vi "Station Detail Main.vi"(8 "error in (no error)":errorcluster, 11 "NG Pick in":refnum<class "NG Pick.lvclass">) -> (0 "error out":errorcluster, 2 "Station Out":T1=enum."ImformOut", 3 "NG Pick out":refnum<class "NG Pick.lvclass">)   [LabVIEW 2019, in "NG Pick.lvclass"]
uses:
  NG Pick.lvclass
  Ctrl/Station Action.ctl
  Ctrl/ProjectStepSelect.ctl
  Ctrl/StationCmdSelect.ctl
  Ctrl/Auto Inspection Station Name2.ctl
  Ctrl/Auto Inspection Data Name.ctl
  Ctrl/MeasureDisplayTab.ctl
  Ctrl/Table Save.ctl
  Ctrl/S2 Station IO.ctl
  Ctrl/ModbusCmd.ctl
  Ctrl/S2 Station Input.ctl
  Global/Process Global.vi
  LLB/Commonly VI/Main Glb.vi
  Ctrl/ProjectCmdStep.ctl
  LineScan/LineScan.lvclass
  LLB/Commonly VI.lvlib
  Ctrl/PD Table Save Low Index.ctl
  Ctrl/PD Table Save Col Index.ctl
panel:
  out "Array":string[](array[string])
  out "Blue Scan receive":string
  out "S1 ChkSum":string
  out "S1 ToolStringOut":string
  out "ToolStringOut_P1_2":string
  out "P1 Receive":string[](array[string])
  out "ToolStringOut_P1":string
  out "ToolStringOut_Init":string
  out "Initial_ChkSum":string
  out "Initial receive 2":string
  in  "Table Control":string[][](table)=[["PCBA BARCODE", ""], ["硬體(Tool初始化)", ""], ["company(Tool初始化)", ""], ["耗電流 uA(電流表)", "T"], ["電池負載電壓", "T"], ["晶片ID(Tool FORMAT)", "F"], ["雷雕ID(TOOl scan、藍芽接收器)", "S"], ["Format(Tool FORMAT)", "F"], ["Programe(Tool Programe)", "P"]]
  out "Numeric":dbl
  out "subarray":string[](array[string])
  out "T2 buffer":string
  out "T1 buffer":string
  out "S2 receive":string
  out "Blue Scan2 receive":string
  out "Program receive":string
  out "format receive":string
  out "Initial receive":string
  out "present":i32
  out "Retry":i32
  out "Act Step":i32
  out "retry次數":string[](array[string])
  out "CurrentCmd":string
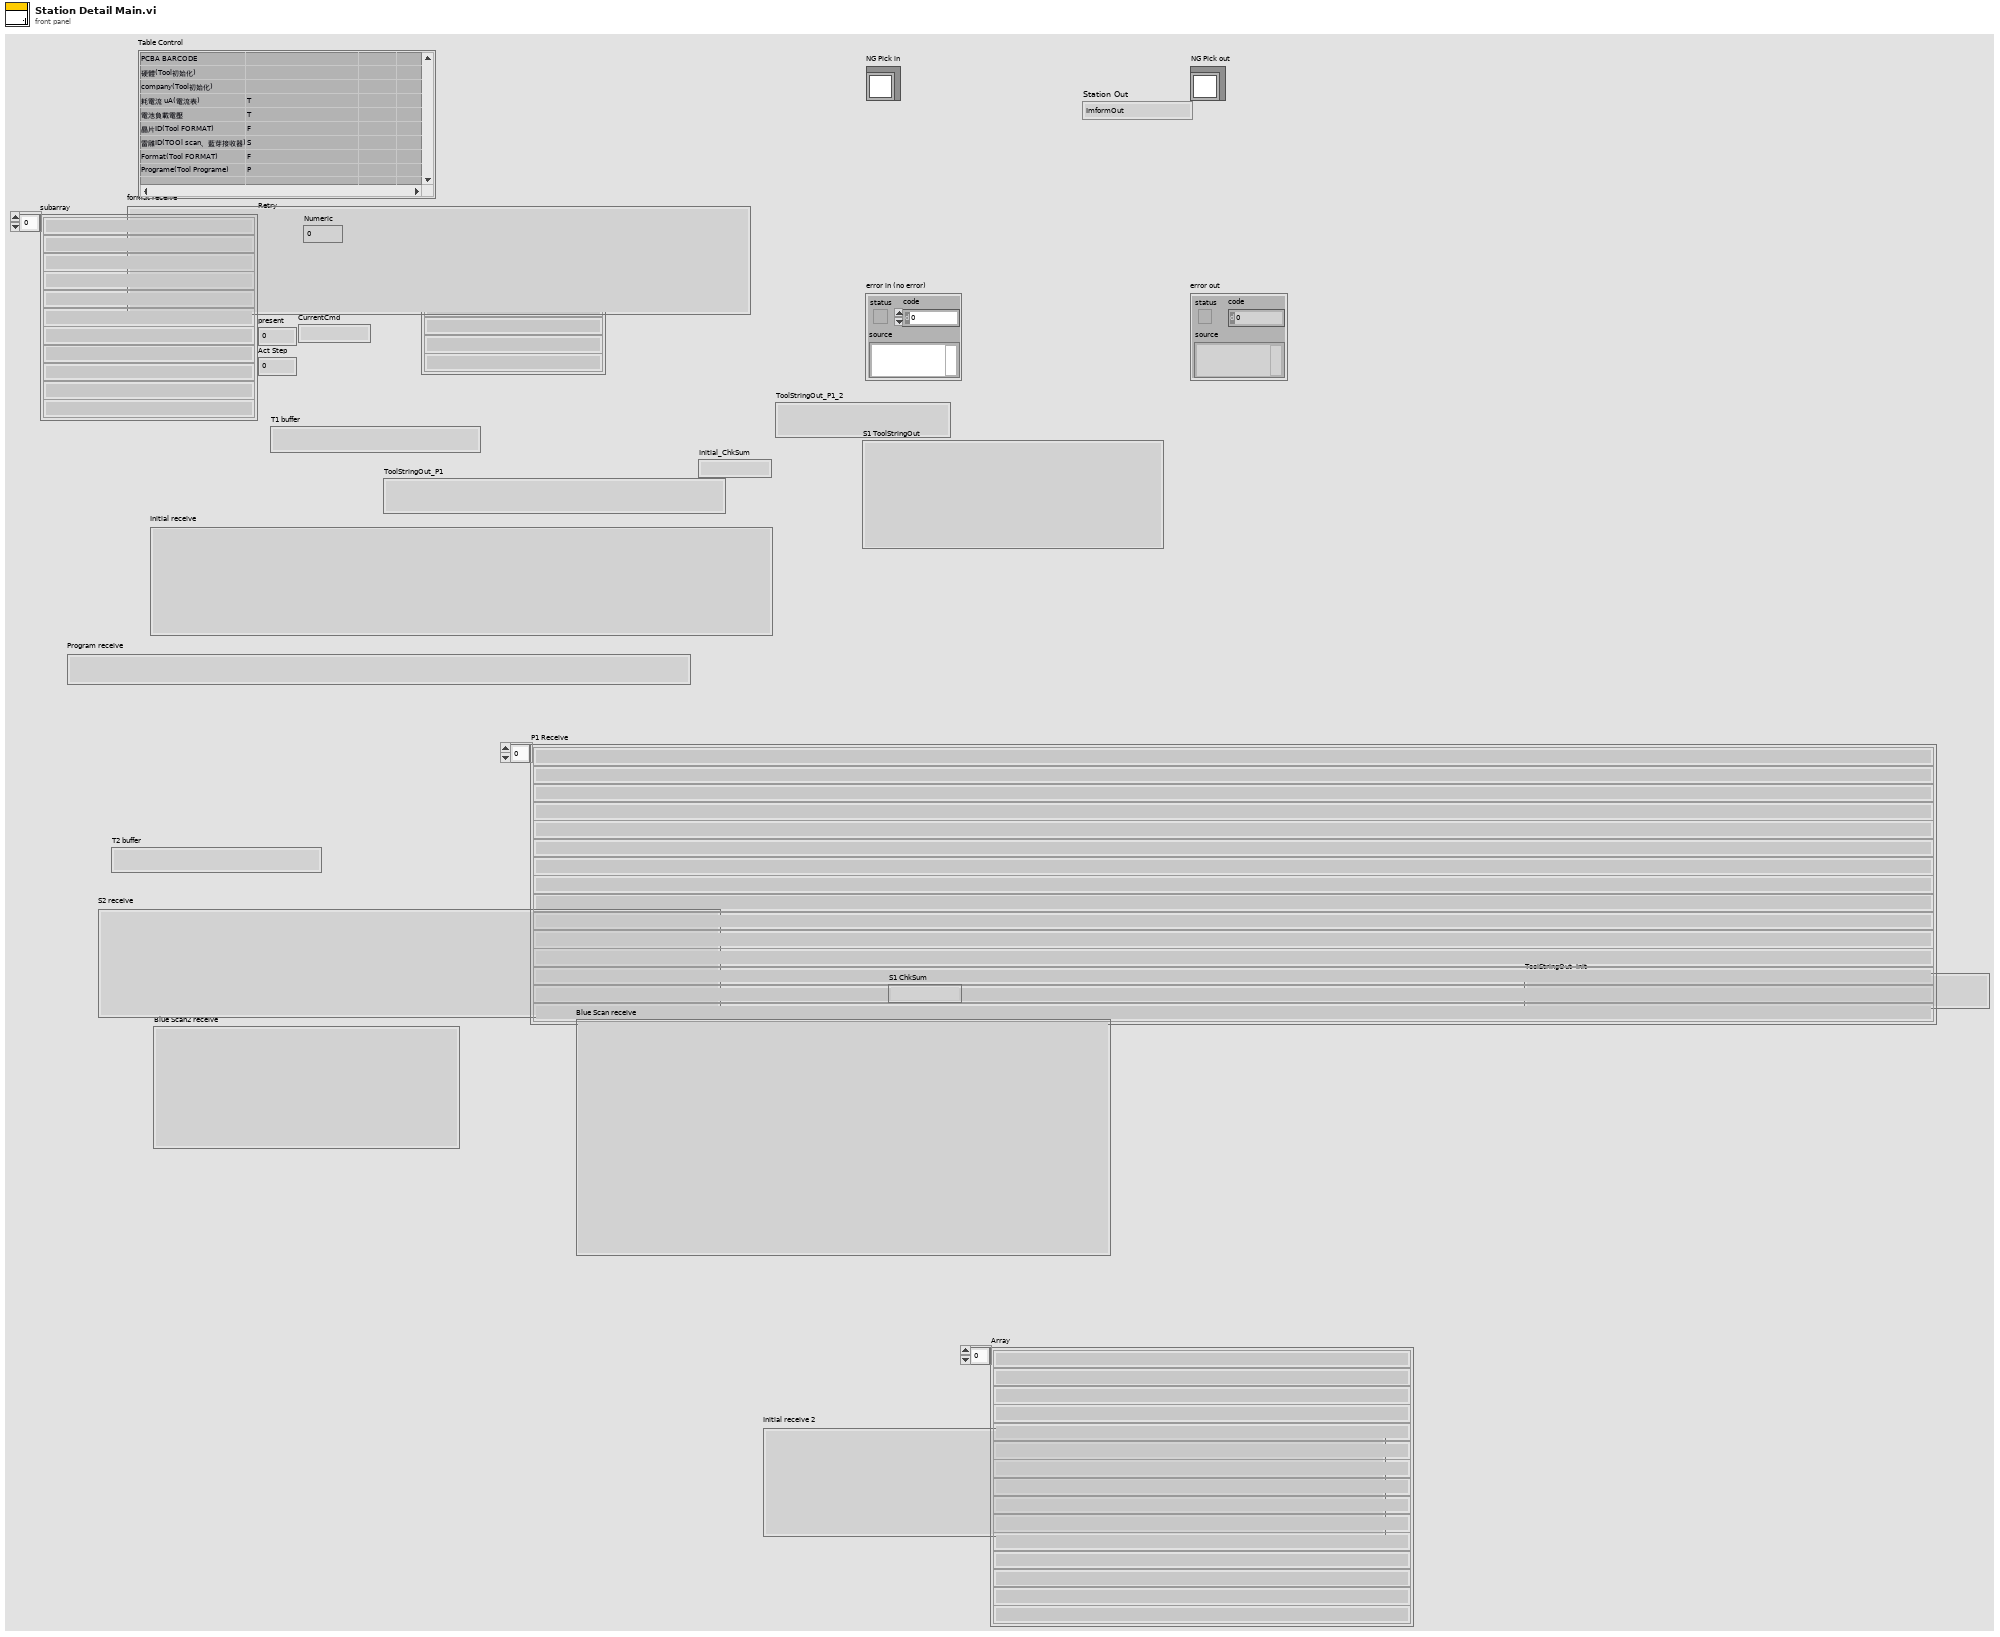
[diagram p1: front panel]
types:
  T1 = typedef "Station Action.ctl" = enum16{"Wait Item In", "Dectect Action", "ImformOut"}
  T2 = typedef "StationCmdSelect.ctl" = enum16{"Action", "Command", "Return", "DTime", "Retry"}
  T3 = typedef "Auto Inspection Data Name.ctl" = enum16{"LocalRun", "ItemSN(TimeCode)", "CurrentAction", "Error", "Data", "OKNG", "電壓值", "電壓值判斷", "電流值", "電流值判斷", "Laser1 Data", "Laser2 Data", "Laser OKNG", "StationNO"}
  T4 = typedef "Auto Inspection Station Name2.ctl" = enum16{"S1Barcode", "S2Measure", "S3Measure", "S4Measure", "S5Measure", "S11_LaserCheck", "S8_Vision AI"}
  T5 = typedef "Table Save.ctl" = enum16{"initial", "Add", "Write", "Replace", "Delete", "REad", "RedTable", "Load"}
  T6 = typedef "MeasureDisplayTab.ctl" = enum16{"Tray Barcode", "PCBA BARCODE", "硬體(Tool初始化)", "company(Tool初始化)", "耗電流 uA(電流表)", "電池負載電壓", "晶片ID(Tool FORMAT)", "雷雕ID(TOOl scan、藍芽接收器)", "Format(Tool FORMAT)", "Programe(Tool Programe)", "MAC(藍芽接收器)", "ID(藍芽接收器)", "KPA(藍芽接收器)", "溫度(藍芽接收器)", "SENSOR電池電壓(藍芽接收器)", "RSSI(藍芽接收器)", "SensorType_315(FSK scan)", "FSKsnVol_315(FSK scan)", "FSKscanl_315(FSK scan)", "P_315(FSK scan)", "T_315(FSK scan)", "SensorType_433(ASK scan)", "ASKsnVol_433(ASK scan)", "ASKscan_433(ASK scan)", "P_433(ASK scan)", "T_433(ASK scan)", "測高Data"}
  T7 = typedef "PD Table Save Col Index.ctl" = enum16{"Col A", "Col B", "PCBA SN_C", "scan 半成品 ID_1_D", "半成品 Waste_Time_E", "半成品 Result_F", "半成品 DateTime_G", "433半成品 版本_H", "433半成品 company_I", "433半成品 FF_J", "433半成品 SensorType_K", "433半成品 BattVol_L", "433半成品 ASKsnVOL_M", "433半成品 ID_2_N", "433半成品 Format_O", "433半成品 Programe_P", "433半成品 ASKscan_Q", "433半成品 FSKscan_R", "433半成品 Batt_S", "433半成品 SN_T", "433半成品 Ptest_U", "433半成品 Ttest_V", "433半成品 P_W", "433半成品 T_X", "433半成品 結果_Y", "433半成品 箱號_Z", "不良代碼_AA", "電流_AB", "電池電壓_AC", "315半成品 版本_AD", "315半成品 company_AE", "315半成品 FF_AF", "315半成品 SensorType_AG", "315半成品 BattVol_AH", "315半成品 ASKsnVOL_AI", "315半成品 ID_2_AJ", "315半成品 Format_AK", "315半成品 Programe_AL", "315半成品 ASKscan_AM", "315半成品 FSKscan_AN", "315半成品 Batt_AO", "315半成品 SN_AP", "315半成品 Ptest_AQ", "315半成品 Ttest_AR", "315半成品 P_AS", "315半成品 T_AT"}
  T8 = typedef "PD Table Save Low Index.ctl" = enum16{"low 1", "low 2", "low 3", "low 4", "一般模式F", "一般模式P", "一般模式S", "low 8", "藍芽模式F", "藍芽模式P", "藍芽模式S"}
  T9 = cluster{"starting address":u16, "number of inputs":u16, "Sat Coils":bool[], "Holding Registers":u16[]}
  T10 = typedef "ModbusCmd.ctl" = enum16{"Connect", "Disconnect", "Init", "Fetch Basic Objects", "Fetch Input Refisters", "Fetch Discrete Inputs", "Set Coils", "Set Holding Registers", "Write Single Holding", "Exit"}
  T11 = typedef "S2 Station Input.ctl" = enum16{"00PLC Alive clock", "01PLC狀態(手動)", "02PLC狀態(自動)", "03PLC Alarm", "04備用", "05備用", "06備用", "07備用", "08備用", "09備用", "10載盤有料for條碼", "11_備用", "12_備用", "13_備用", "14_備用", "15_備用", "16_備用", "17_備用", "18_備用", "19_備用", "20_載盤有料訊號ForS2站", "21_PLC下達可測電流訊號", "22_PLC下達可測電壓訊號"}
  T12 = typedef "ProjectStepSelect.ctl" = enum16{"ProjectName", "Name", "Initial", "Reset", "Format", "Program1", "Program2", "Scan", "Finish", "MToolWork", "DataCheck", "DataSave", "OutputPLC", "WaitInputS1", "WaitInputOff"}
  T13 = typedef "S2 Station IO.ctl" = enum16{"S2站PC動作中_20", "電流量測完成產品OK_21", "電流量測完成產品NG_22", "S2站Format 執行_23", "S2 Format OK_24", "S2 Format NG_25", "S2站燒入執行_26", "S2站燒入OK_27", "S2站燒入NG_28", "S2站動作完成_29", "S3 PC動作中_30", "S3 Format 此站執行_31", "S3 Format OK_32", "S3 Format NG_33", "S3 燒入程式 此站執行_34", "S3 燒入程式 OK_35", "S3 燒入程式 NG_36", "S3 備用_37", "S3 備用_38", "S3 動作完成_39", "S4 PC動作中_40", "S4 量測完成 產品正常_41", "S4 量測完成 產品NG_42", "S4 Format 此站執行_43", "S4 Format OK_44", "S4 Format NG_45", "S4 燒入 此站不執行_46", "S4 燒入程式 OK_47", "S4 燒入程式 NG_48", "S4 藍芽Scan OK_49", "S4 藍芽Scan NG_50", "S4 動作完成_51", "給PLC要量電流訊號", "給PLC要量電壓訊號"}
  T14 = typedef "ProjectCmdStep.ctl" = enum16{"Project Name", "commamd1", "commamd2", "commamd3", "wat time1", "return1", "return2", "return3", "wat time2", "over time", "retry"}
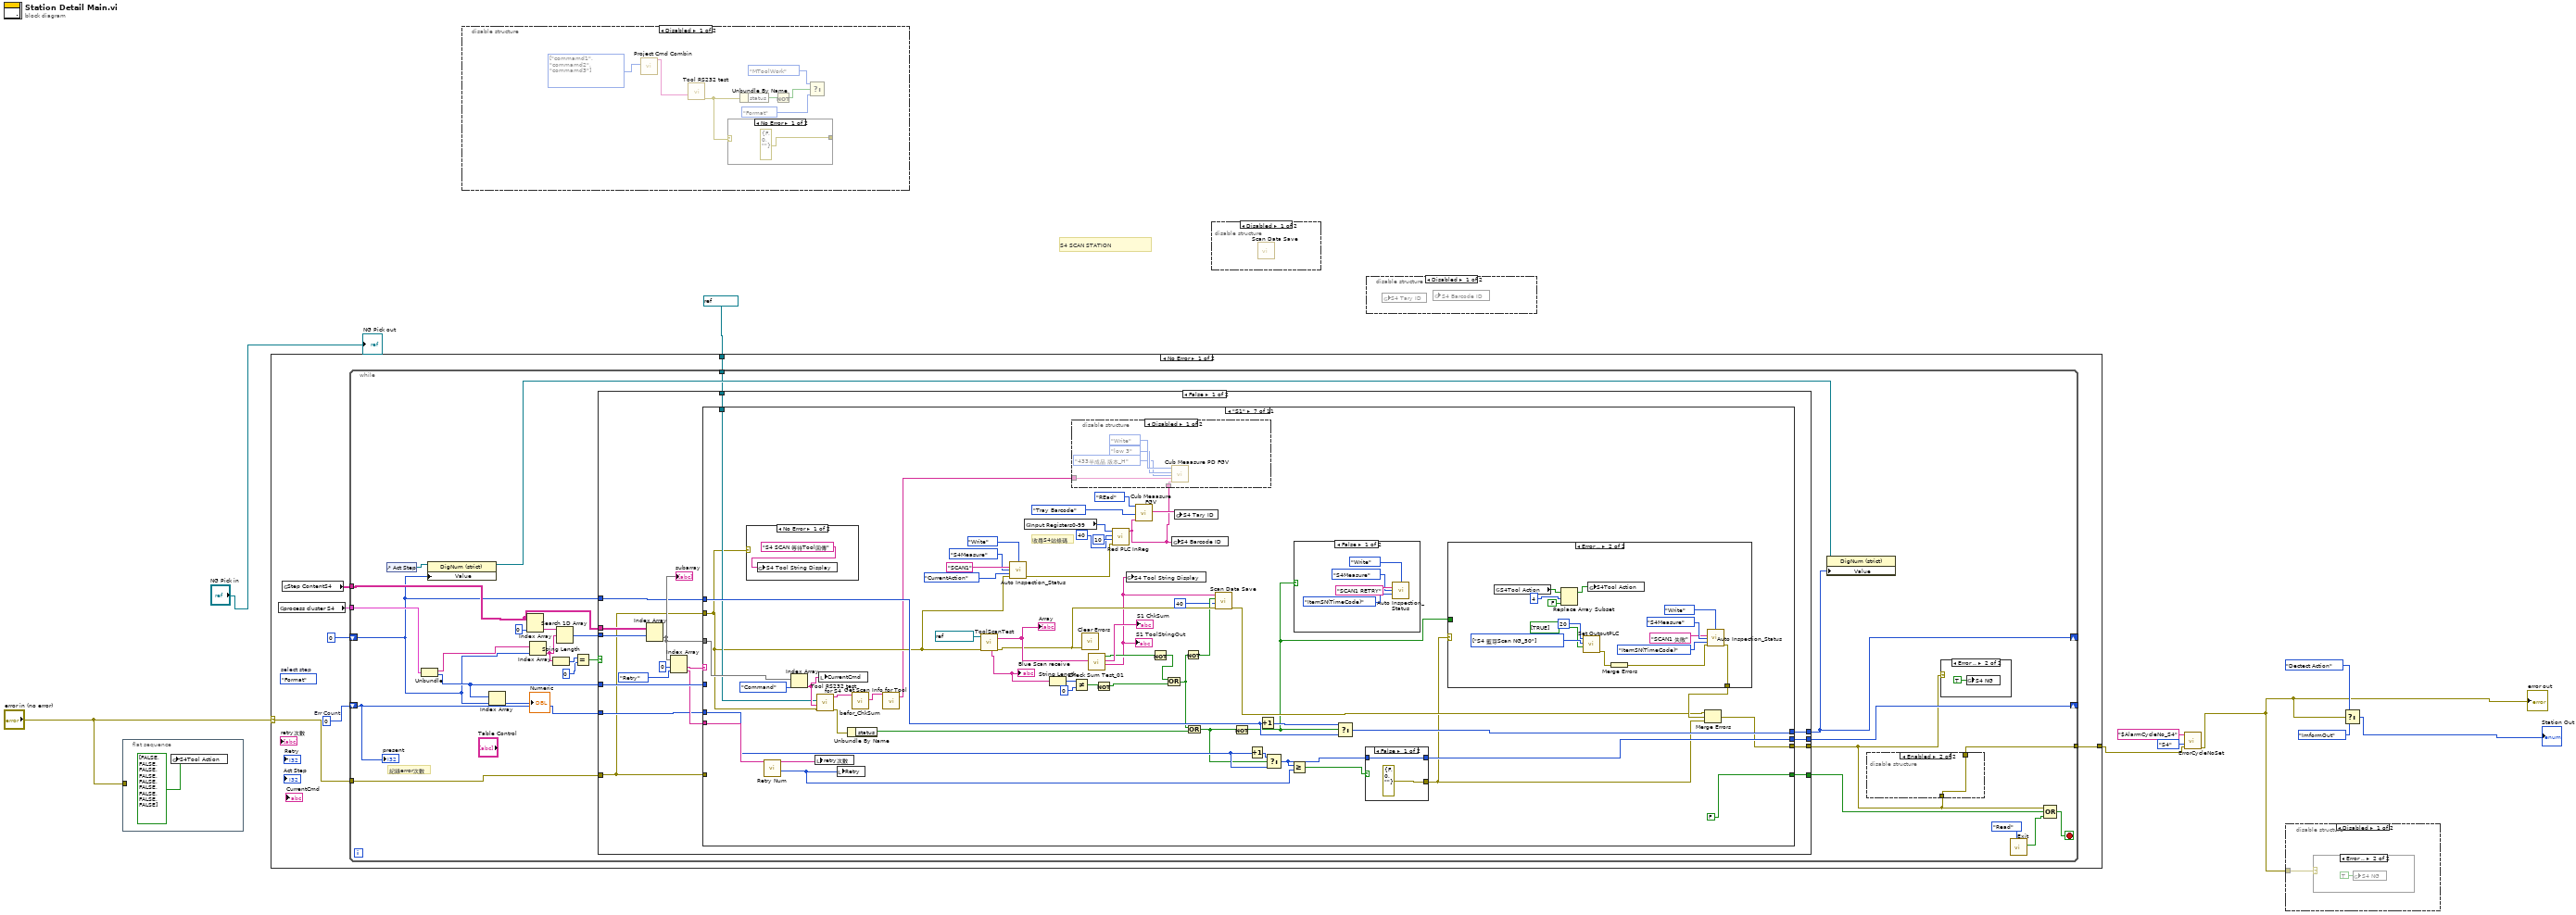
[diagram p0: block diagram]
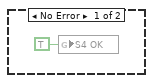
[diagram p2: hidden frame]
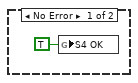
[diagram p6: hidden frame]
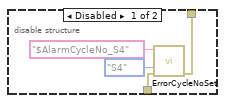
[diagram p7: hidden frame]
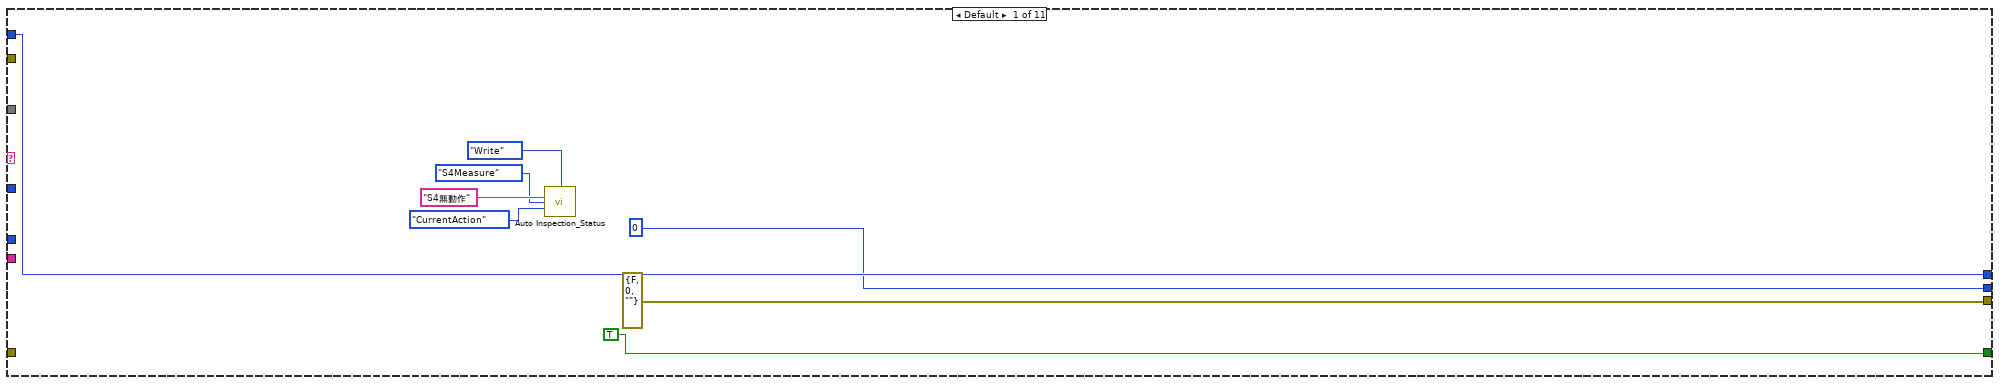
[diagram p8: hidden frame]
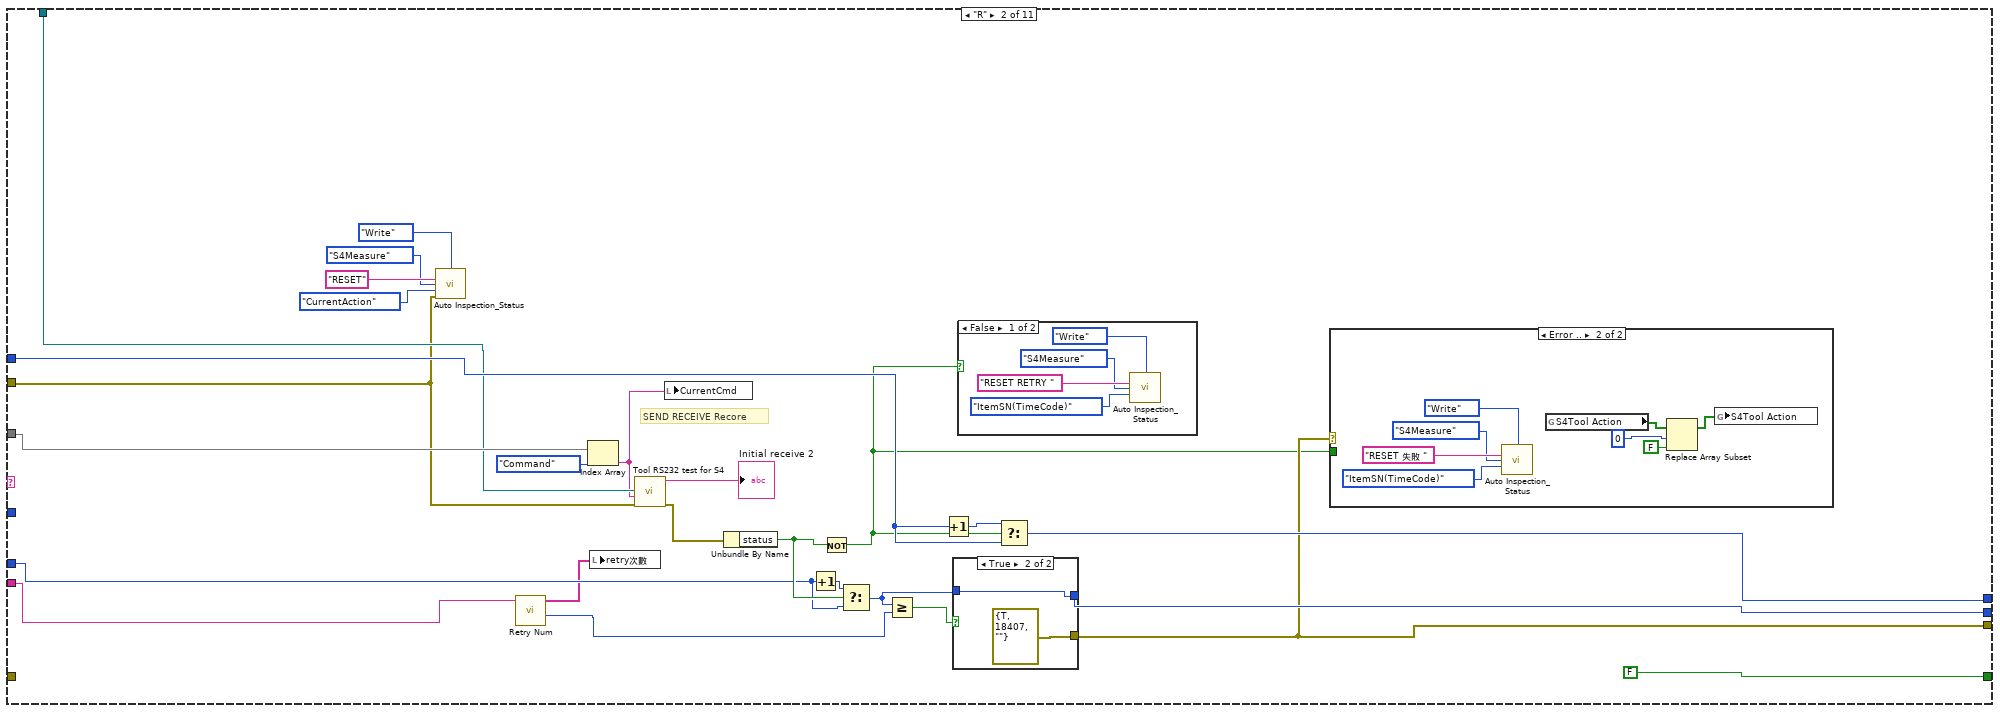
[diagram p9: hidden frame]
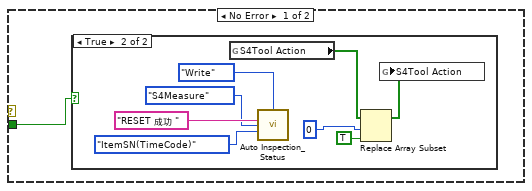
[diagram p11: hidden frame]
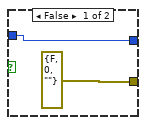
[diagram p13: hidden frame]
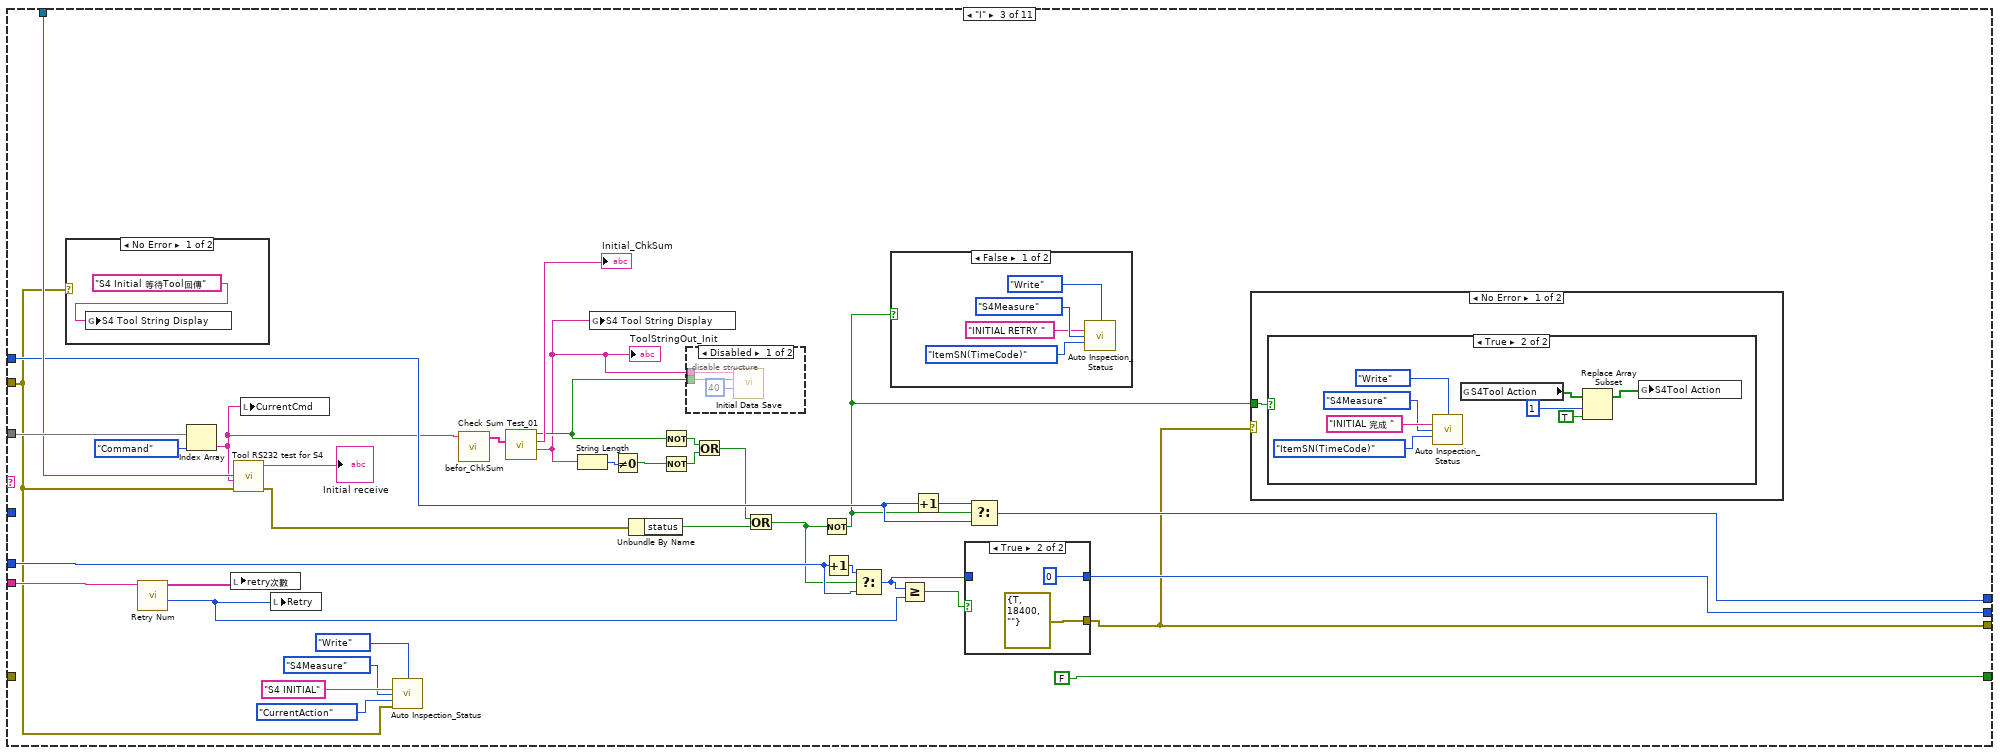
[diagram p14: hidden frame]
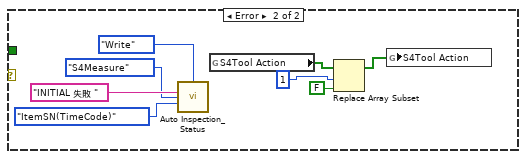
[diagram p19: hidden frame]
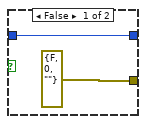
[diagram p20: hidden frame]
diagram:
  # "S4 SCAN STATION"
  n1 = flat-sequence {
    tunnel: "error in (no error)" -> [_]
    frame #0 {
      n2 = global write "Process Global.vi" "S4Tool Action"(bool[] [FALSE, FALSE, FALSE, FALSE, FALSE, FALSE, FALSE, FALSE, FALSE] ("S4Tool Action")) -> ()
    }
  }
  n3 = case shown="No Error" "error in (no error)" {
    selector: "error in (no error)" -> [w13 w807]
    tunnel: [w18 w807] -> w2
    tunnel: refnum<visa-resource-name> "COM2" ("VISA resource name") -> [w12 _]
    frame No Error {
      w14 = 0  # Err Count
      (unwired) ProjectStepSelect."Format"  # select step
      n4 = global read "Process Global.vi" "process cluster S4"() -> (w16:cluster{string[], i32[]})
      n5 = global read "Process Global.vi" "Step ContentS4"() -> (w17:string[][])
      n6 = while {
        tunnel: [w20] -> w18
        shift-right: [w26] -> _
        shift-left: 0 -> [w27]
        shift-right: [w29] -> _
        shift-left: w14 -> [w30]
        tunnel: w17 -> [w41]
        tunnel: w16 -> [w40]
        tunnel: w13 -> [w24]
        tunnel: w12 -> [w23]
        stop <- w42 stop-if-true
        # "紀錄error次數"
        n7 = control-ref of="Act Step"() -> (w28:refnum<vi>)
        n8 = Unbundle(w40) -> (w43:string[], w44:i32[])
        n9 = property class="DigNum (strict)"(reference=w28, "Value"=w27) -> (reference out=w25:refnum<vi>)  [unwired: 1 in, 1 out]
        n10 = Index Array(array=w44, index=w27) -> (element=→"Numeric":i32)
        n11 = Index Array(array=w41, index (col)=0 ("disabled index (col)")) -> (element=w38:string[])  [unwired: 1 in]
        n12 = Index Array(array=w43, index=w27) -> (element=w34:string)
        n13 = String Length(string=w34) -> (length=w35:i32)
        n14 = Search 1D Array(1D array=w38, element=w34) -> (index of element=w37:i32)  [unwired: 1 in]
        n15 = Equal?(x=w35, y=0) -> (x = y?=w32:bool)
        n16 = case shown="False" w32 {
          tunnel: w44 -> [w67 _]
          tunnel: w41 -> [w66 _]
          tunnel: w37 -> [w65 _]
          tunnel: [w54 TRUE] -> w31
          tunnel: [w57 errorcluster {"status"=FALSE, "code"=0, "source"=""} ("error constant")] -> w19
          tunnel: w27 -> [w60 _]
          tunnel: [w59 0] -> w26
          tunnel: w30 -> [w58 _]
          tunnel: [w56 0 ("Err Count")] -> w29
          tunnel: w24 -> [w53 _]
          tunnel: w23 -> [w52 _]
          frame False {
            n17 = Index Array(array=w66, index (row)=w65) -> (element=w61:string[])  [unwired: 1 in]
            "subarray" <- w61
            n18 = Index Array(array=w61, index #1=0 ("index"), index #2=StationCmdSelect."Retry") -> (element #1=w63:string, element #2=w62:string)
            n19 = case shown="\"S1\"" w63 {
              tunnel: w67 -> [_ _ _ _ _ _ _ _ w584 _ _]
              tunnel: w62 -> [_ w85 w151 w226 w323 _ w431 w535 _ w598 w705]
              tunnel: w61 -> [_ w88 w153 w225 w325 _ w430 w536 _ _ _]
              tunnel: w60 -> [w75 w87 w142 w221 w324 w386 w429 w537 w579 w596 w707]
              tunnel: [w75 w81 w149 w223 w320 w385 w433 w533 w578 w595 w706] -> w59
              tunnel: w58 -> [_ w84 w152 w217 w322 _ w428 w534 _ w599 w704]
              tunnel: [errorcluster {"status"=FALSE, "code"=0, "source"=""} ("error constant") w78 w129 w207 w289 errorcluster {"status"=FALSE, "code"=0, "source"=""} ("error IO") w418 w531 errorcluster {"status"=FALSE, "code"=0, "source"=""} ("error constant") w594 w703] -> w57
              tunnel: [0 ("Err Count") w83 w150 w212 w321 0 ("Err Count") w432 w532 0 ("Err Count") w597 w708] -> w56
              tunnel: [TRUE FALSE FALSE FALSE FALSE FALSE FALSE FALSE FALSE FALSE FALSE] -> w54
              tunnel: w53 -> [_ _ _ _ _ _ _ _ _ _ _]
              tunnel: w53 -> [_ w77 w128 w192 w279 _ w400 w486 _ _ _]
              tunnel: w52 -> [_ w86 w143 w202 w297 _ w419 w530 _ _ _]
              frame Default {
                n20 = call "Auto Inspection_Status.vi"("Action"=enum16{"Initial", "Write", "Read"}."Write", "DataIn"="S4無動作", "Station"=Auto_Inspection_Station_Name2."S4Measure", "Data"=Auto_Inspection_Data_Name."CurrentAction") -> ()  [unwired: 9 in, 3 out]
              }
              frame "R" {
                # "SEND RECEIVE Recore"
                n21 = call "Auto Inspection_Status.vi"("Action"=enum16{"Initial", "Write", "Read"}."Write", "DataIn"="RESET", "Station"=Auto_Inspection_Station_Name2."S4Measure", "Data"=Auto_Inspection_Data_Name."CurrentAction", "error in"=w77) -> ()  [unwired: 8 in, 3 out]
                n22 = call "Retry Num.vi"("String"=w85) -> ("Numeric"=w99:i32, "retry次數"=w80:string[])  [unwired: 9 in]
                n23 = Index Array(array=w88, index=StationCmdSelect."Command") -> (element=w79:string)
                n24 = local write "retry次數"(w80) -> ()
                n25 = call "Tool RS232 test for S4.vi"("error in (no error)"=w77, "Cmd In"=w79, "VISA resource name"=w86) -> ("error out"=w95:errorcluster, "receive string"=→"Initial receive 2":string)  [unwired: 7 in]
                n26 = local write "CurrentCmd"(w79) -> ()
                n27 = Unbundle By Name(w95) -> ("status"=w97:bool)
                n28 = Increment(x=w84) -> (x+1=w98:i32)
                n29 = Not(x=w97) -> (.not. x?=w76:bool)
                n30 = Select(t=w98, s=w97, f=w84) -> (s? t:f=w100:i32)
                n31 = Greater Or Equal?(x=w100, y=w99) -> (x >= y?=w101:bool)
                n32 = Increment(x=w87) -> (x+1=w96:i32)
                n33 = case shown="True" w101 {
                  tunnel: [errorcluster {"status"=FALSE, "code"=0, "source"=""} ("error constant") errorcluster {"status"=TRUE, "code"=18407, "source"=""} ("error constant")] -> w78
                  tunnel: w100 -> [w123 w125]
                  tunnel: [w123 w125] -> w83
                  frame False {
                  }
                  frame True {
                  }
                }
                n34 = case shown="False" w76 {
                  frame False {
                    n35 = call "Auto Inspection_Status.vi"("Action"=enum16{"Initial", "Write", "Read"}."Write", "DataIn"="RESET RETRY ", "Station"=Auto_Inspection_Station_Name2."S4Measure", "Data"=Auto_Inspection_Data_Name."ItemSN(TimeCode)") -> ()  [unwired: 9 in, 3 out]
                  }
                  frame True {
                  }
                }
                n36 = Select(t=w96, s=w76, f=w87) -> (s? t:f=w81:i32)
                n37 = case shown="Error .." w78 {
                  tunnel: w76 -> [w106 _]
                  frame No Error {
                    n38 = case shown="True" w106 {
                      frame False {
                      }
                      frame True {
                        n39 = global read "Process Global.vi" "S4Tool Action"() -> (w110:bool[])
                        n40 = call "Auto Inspection_Status.vi"("Action"=enum16{"Initial", "Write", "Read"}."Write", "DataIn"="RESET 成功 ", "Station"=Auto_Inspection_Station_Name2."S4Measure", "Data"=Auto_Inspection_Data_Name."ItemSN(TimeCode)") -> ()  [unwired: 9 in, 3 out]
                        n41 = Replace Array Subset(array=w110, new element=TRUE ("new element/subarray"), index=0) -> (w107:bool[])
                        n42 = global write "Process Global.vi" "S4Tool Action"(w107) -> ()
                      }
                    }
                  }
                  frame Error {
                    n43 = call "Auto Inspection_Status.vi"("Action"=enum16{"Initial", "Write", "Read"}."Write", "DataIn"="RESET 失敗 ", "Station"=Auto_Inspection_Station_Name2."S4Measure", "Data"=Auto_Inspection_Data_Name."ItemSN(TimeCode)") -> ()  [unwired: 9 in, 3 out]
                    n44 = global read "Process Global.vi" "S4Tool Action"() -> (w118:bool[])
                    n45 = Replace Array Subset(array=w118, new element=FALSE ("new element/subarray"), index=0) -> (w115:bool[])
                    n46 = global write "Process Global.vi" "S4Tool Action"(w115) -> ()
                  }
                }
              }
              frame "I" {
                n47 = case shown="No Error" w128 {
                  frame No Error {
                    n48 = global write "Process Global.vi" "S4 Tool String Display"("S4 Initial 等待Tool回傳") -> ()
                  }
                  frame Error {
                  }
                }
                n49 = call "Retry Num.vi"("String"=w151) -> ("Numeric"=w158:i32, "retry次數"=w155:string[])  [unwired: 9 in]
                n50 = Index Array(array=w153, index=StationCmdSelect."Command") -> (element=w135:string)
                n51 = local write "retry次數"(w155) -> ()
                n52 = call "Tool RS232 test for S4.vi"("error in (no error)"=w128, "Cmd In"=w135, "VISA resource name"=w143) -> ("error out"=w161:errorcluster, "receive string"=→"Initial receive":string)  [unwired: 7 in]
                n53 = local write "CurrentCmd"(w135) -> ()
                n54 = local write "Retry"(w158) -> ()
                n55 = call "Auto Inspection_Status.vi"("Action"=enum16{"Initial", "Write", "Read"}."Write", "DataIn"="S4 INITIAL", "Station"=Auto_Inspection_Station_Name2."S4Measure", "Data"=Auto_Inspection_Data_Name."CurrentAction", "error in"=w128) -> ()  [unwired: 8 in, 3 out]
                n56 = call "befor_ChkSum.vi"("ToolString Input"=w135) -> ("Array"=w140:string[])  [unwired: 9 in, 1 out]
                n57 = call "Check Sum Test_01.vi"("Array"=w140) -> ("ToolStringOut_01"=w130:string, "ChkSum"=→"Initial_ChkSum":string, "x = y?"=w131:bool)  [unwired: 8 in]
                "ToolStringOut_Init" <- w130
                n58 = String Length(string=w130) -> (length=w137:i32)
                n59 = global write "Process Global.vi" "S4 Tool String Display"(w130) -> ()
                n60 = Not Equal To 0?(x=w137) -> (x != 0?=w136:bool)
                n61 = Unbundle By Name(w161) -> ("status"=w134:bool)
                n62 = Not(x=w131) -> (.not. x?=w139:bool)
                n63 = Not(x=w136) -> (.not. x?=w138:bool)
                n64 = disable-structure shown="Disabled" {
                  disable-tunnel: w131 -> [w170 _]
                  disable-tunnel: w130 -> [w168 _]
                  frame Disabled {
                    n65 = call "Initial Data Save.vi"("index"=40, "OK and NG"=w170, "String In"=w168) -> ()  [unwired: 8 in, 1 out]
                  }
                  frame Enabled {
                  }
                }
                n66 = Or(x=w139, y=w138) -> (x .or. y?=w133:bool)
                n67 = Or(x=w133, y=w134) -> (x .or. y?=w132:bool)
                n68 = Not(x=w132) -> (.not. x?=w127:bool)
                n69 = Increment(x=w152) -> (x+1=w159:i32)
                n70 = Select(t=w159, s=w132, f=w152) -> (s? t:f=w156:i32)
                n71 = case shown="False" w127 {
                  frame False {
                    n72 = call "Auto Inspection_Status.vi"("Action"=enum16{"Initial", "Write", "Read"}."Write", "DataIn"="INITIAL RETRY ", "Station"=Auto_Inspection_Station_Name2."S4Measure", "Data"=Auto_Inspection_Data_Name."ItemSN(TimeCode)") -> ()  [unwired: 9 in, 3 out]
                  }
                  frame True {
                  }
                }
                n73 = Greater Or Equal?(x=w156, y=w158) -> (x >= y?=w157:bool)
                n74 = Increment(x=w142) -> (x+1=w160:i32)
                n75 = case shown="True" w157 {
                  tunnel: [errorcluster {"status"=FALSE, "code"=0, "source"=""} ("error constant") errorcluster {"status"=TRUE, "code"=18400, "source"=""} ("error constant")] -> w129
                  tunnel: w156 -> [w188 _]
                  tunnel: [w188 0] -> w150
                  frame False {
                  }
                  frame True {
                  }
                }
                n76 = Select(t=w160, s=w127, f=w142) -> (s? t:f=w149:i32)
                n77 = case shown="No Error" w129 {
                  tunnel: w127 -> [w171 _]
                  frame No Error {
                    n78 = case shown="True" w171 {
                      frame False {
                      }
                      frame True {
                        n79 = call "Auto Inspection_Status.vi"("Action"=enum16{"Initial", "Write", "Read"}."Write", "DataIn"="INITIAL 完成 ", "Station"=Auto_Inspection_Station_Name2."S4Measure", "Data"=Auto_Inspection_Data_Name."ItemSN(TimeCode)") -> ()  [unwired: 9 in, 3 out]
                        n80 = global read "Process Global.vi" "S4Tool Action"() -> (w173:bool[])
                        n81 = Replace Array Subset(array=w173, new element=TRUE ("new element/subarray"), index=1) -> (w172:bool[])
                        n82 = global write "Process Global.vi" "S4Tool Action"(w172) -> ()
                      }
                    }
                  }
                  frame Error {
                    n83 = call "Auto Inspection_Status.vi"("Action"=enum16{"Initial", "Write", "Read"}."Write", "DataIn"="INITIAL 失敗 ", "Station"=Auto_Inspection_Station_Name2."S4Measure", "Data"=Auto_Inspection_Data_Name."ItemSN(TimeCode)") -> ()  [unwired: 9 in, 3 out]
                    n84 = global read "Process Global.vi" "S4Tool Action"() -> (w183:bool[])
                    n85 = Replace Array Subset(array=w183, new element=FALSE ("new element/subarray"), index=1) -> (w180:bool[])
                    n86 = global write "Process Global.vi" "S4Tool Action"(w180) -> ()
                  }
                }
              }
              frame "F" {
                # "收尋S4站條碼"
                # "SEND RECEIVE Recore"
                n87 = call "Retry Num.vi"("String"=w226) -> ("Numeric"=w216:i32, "retry次數"=w211:string[])  [unwired: 9 in]
                n88 = Index Array(array=w225, index=StationCmdSelect."Command") -> (element=w210:string)
                n89 = local write "Retry"(w216) -> ()
                n90 = local write "retry次數"(w211) -> ()
                n91 = call "Tool RS232 test for S4.vi"("error in (no error)"=w192, "Cmd In"=w210, "VISA resource name"=w202) -> ("error out"=w222:errorcluster, "receive string"=→"format receive":string)  [unwired: 7 in]
                n92 = local write "CurrentCmd"(w210) -> ()
                n93 = call "Auto Inspection_Status.vi"("Action"=enum16{"Initial", "Write", "Read"}."Write", "DataIn"="FORMAT", "Station"=Auto_Inspection_Station_Name2."S4Measure", "Data"=Auto_Inspection_Data_Name."CurrentAction", "error in"=w192) -> ()  [unwired: 8 in, 3 out]
                n94 = Unbundle By Name(w222) -> ("status"=w219:bool)
                n95 = global read "Main Glb.vi" "Input Registers0-99"() -> (w198:u16[])
                n96 = Not(x=w219) -> (.not. x?=w200:bool)
                n97 = Increment(x=w217) -> (x+1=w218:i32)
                n98 = Select(t=w218, s=w219, f=w217) -> (s? t:f=w213:i32)
                n99 = Greater Or Equal?(x=w213, y=w216) -> (x >= y?=w215:bool)
                n100 = call "Red PLC InReg.vi"("error in (no error)"=w192, "length"=10, "index"=40, "Input Registers Arr"=w198) -> ("Rad In Reg"=w194:string)  [unwired: 6 in, 1 out]
                n101 = call "Cub Meaasure FGV.vi"("Action"=Table_Save."REad" ("Enum"), "Save Index"=MeasureDisplayTab."Tray Barcode", "SN"=w194) -> ("Read Index Data"=w193:string)  [unwired: 9 in, 7 out]
                n102 = case shown="True" w215 {
                  tunnel: [errorcluster {"status"=FALSE, "code"=0, "source"=""} ("error constant") errorcluster {"status"=TRUE, "code"=18401, "source"=""} ("error constant")] -> w201
                  tunnel: w213 -> [w275 _]
                  tunnel: [w275 0] -> w212
                  frame False {
                  }
                  frame True {
                  }
                }
                n103 = global write "Main Glb.vi" "S4 Barcode ID"(w194) -> ()
                n104 = global write "Main Glb.vi" "S4 Tary ID"(w193) -> ()
                n105 = case shown="False" w200 {
                  frame False {
                    n106 = call "Auto Inspection_Status.vi"("Action"=enum16{"Initial", "Write", "Read"}."Write", "DataIn"="FORMAT RETRY ", "Station"=Auto_Inspection_Station_Name2."S4Measure", "Data"=Auto_Inspection_Data_Name."ItemSN(TimeCode)") -> ()  [unwired: 9 in, 3 out]
                  }
                  frame True {
                    n107 = call "Auto Inspection_Status.vi"("Action"=enum16{"Initial", "Write", "Read"}."Write", "DataIn"="FORMAT完成", "Station"=Auto_Inspection_Station_Name2."S4Measure", "Data"=Auto_Inspection_Data_Name."ItemSN(TimeCode)") -> ()  [unwired: 9 in, 3 out]
                  }
                }
                n108 = Increment(x=w221) -> (x+1=w220:i32)
                n109 = Select(t=w220, s=w200, f=w221) -> (s? t:f=w223:i32)
                n110 = case shown="Error .." w201 {
                  tunnel: [w236 w272] -> w208
                  tunnel: w200 -> [w235 _]
                  frame No Error {
                    n111 = case shown="True" w235 {
                      tunnel: [_ w253] -> w236
                      frame False {
                      }
                      frame True {
                        w254 = T13[] [enum."S4 Format 此站執行_43", enum."S4 Format OK_44"] items=["S2站PC動作中_20", "電流量測完成產品OK_21", "電流量測完成產品NG_22", "S2站Format 執行_23", "S2 Format OK_24", "S2 Format NG_25", "S2站燒入執行_26", "S2站燒入OK_27", "S2站燒入NG_28", "S2站動作完成_29", "S3 PC動作中_30", "S3 Format 此站執行_31", "S3 Format OK_32", "S3 Format NG_33", "S3 燒入程式 此站執行_34", "S3 燒入程式 OK_35", "S3 燒入程式 NG_36", "S3 備用_37", "S3 備用_38", "S3 動作完成_39", "S4 PC動作中_40", "S4 量測完成 產品正常_41", "S4 量測完成 產品NG_42", "S4 Format 此站執行_43", "S4 Format OK_44", "S4 Format NG_45", "S4 燒入 此站不執行_46", "S4 燒入程式 OK_47", "S4 燒入程式 NG_48", "S4 藍芽Scan OK_49", "S4 藍芽Scan NG_50", "S4 動作完成_51", "給PLC要量電流訊號", "給PLC要量電壓訊號"]
                        # "收尋S4站條碼"
                        n112 = global read "Main Glb.vi" "Input Registers0-99"() -> (w242:u16[])
                        n113 = global read "Process Global.vi" "S4Tool Action"() -> (w248:bool[])
                        n114 = call "Set OutputPLC.vi"("Address In"=20, "Array 2"=w254, "Sat Coils"=bool[] [TRUE]) -> ("Error Out"=w253:errorcluster[])  [unwired: 7 in]
                        n115 = call "Red PLC InReg.vi"("length"=10, "index"=40, "Input Registers Arr"=w242) -> ("Rad In Reg"=w245:string)  [unwired: 7 in, 1 out]
                        n116 = Replace Array Subset(array=w248, new element=TRUE ("new element/subarray"), index=2) -> (w238:bool[])
                        n117 = call "Cub Meaasure FGV.vi"("Action"=Table_Save."Write" ("Enum"), "Save Index"=MeasureDisplayTab."Format(Tool FORMAT)", "DataIn"="OK", "SN"=w245) -> ()  [unwired: 8 in, 8 out]
                        n118 = global write "Process Global.vi" "S4Tool Action"(w238) -> ()
                        n119 = call "Auto Inspection_Status.vi"("Action"=enum16{"Initial", "Write", "Read"}."Write", "DataIn"="FORMAT完成", "Station"=Auto_Inspection_Station_Name2."S4Measure", "Data"=Auto_Inspection_Data_Name."ItemSN(TimeCode)") -> ()  [unwired: 9 in, 3 out]
                      }
                    }
                  }
                  frame Error {
                    w274 = T13[] [enum."S4 Format 此站執行_43", enum."S4 Format NG_45"] items=["S2站PC動作中_20", "電流量測完成產品OK_21", "電流量測完成產品NG_22", "S2站Format 執行_23", "S2 Format OK_24", "S2 Format NG_25", "S2站燒入執行_26", "S2站燒入OK_27", "S2站燒入NG_28", "S2站動作完成_29", "S3 PC動作中_30", "S3 Format 此站執行_31", "S3 Format OK_32", "S3 Format NG_33", "S3 燒入程式 此站執行_34", "S3 燒入程式 OK_35", "S3 燒入程式 NG_36", "S3 備用_37", "S3 備用_38", "S3 動作完成_39", "S4 PC動作中_40", "S4 量測完成 產品正常_41", "S4 量測完成 產品NG_42", "S4 Format 此站執行_43", "S4 Format OK_44", "S4 Format NG_45", "S4 燒入 此站不執行_46", "S4 燒入程式 OK_47", "S4 燒入程式 NG_48", "S4 藍芽Scan OK_49", "S4 藍芽Scan NG_50", "S4 動作完成_51", "給PLC要量電流訊號", "給PLC要量電壓訊號"]
                    # "收尋S4站條碼"
                    n120 = global read "Main Glb.vi" "Input Registers0-99"() -> (w259:u16[])
                    n121 = call "Set OutputPLC.vi"("Address In"=20, "Array 2"=w274, "Sat Coils"=bool[] [TRUE]) -> ("Error Out"=w272:errorcluster[])  [unwired: 7 in]
                    n122 = global read "Process Global.vi" "S4Tool Action"() -> (w266:bool[])
                    n123 = call "Red PLC InReg.vi"("length"=10, "index"=40, "Input Registers Arr"=w259) -> ("Rad In Reg"=w262:string)  [unwired: 7 in, 1 out]
                    n124 = Replace Array Subset(array=w266, new element=FALSE ("new element/subarray"), index=2) -> (w263:bool[])
                    n125 = call "Cub Meaasure FGV.vi"("Action"=Table_Save."Write" ("Enum"), "Save Index"=MeasureDisplayTab."Format(Tool FORMAT)", "DataIn"="NG", "SN"=w262) -> ()  [unwired: 8 in, 8 out]
                    n126 = global write "Process Global.vi" "S4Tool Action"(w263) -> ()
                    n127 = call "Auto Inspection_Status.vi"("Action"=enum16{"Initial", "Write", "Read"}."Write", "DataIn"="FORMAT 失敗 ", "Station"=Auto_Inspection_Station_Name2."S4Measure", "Data"=Auto_Inspection_Data_Name."ItemSN(TimeCode)") -> ()  [unwired: 9 in, 3 out]
                  }
                }
                n128 = Merge Errors(w208, w201) -> (w207:errorcluster)
              }
              frame "P1" {
                # "收尋S4站條碼"
                # "經過燒錄後第二次Tool回傳"
                # "下Cmd後第一次Tool回傳"
                n129 = call "Retry Num.vi"("String"=w323) -> ("Numeric"=w330:i32, "retry次數"=w327:string[])  [unwired: 9 in]
                n130 = Index Array(array=w325, index=StationCmdSelect."Command") -> (element=w296:string)
                n131 = local write "retry次數"(w327) -> ()
                n132 = local write "Retry"(w330) -> ()
                n133 = call "Tool RS232 test for S4.vi"("error in (no error)"=w279, "Cmd In"=w296, "VISA resource name"=w297) -> ("error out"=w294:errorcluster, "receive string"=→"Program receive":string)  [unwired: 7 in]
                n134 = call "Auto Inspection_Status.vi"("Action"=enum16{"Initial", "Write", "Read"}."Write", "DataIn"="PROGRAM1", "Station"=Auto_Inspection_Station_Name2."S4Measure", "Data"=Auto_Inspection_Data_Name."CurrentAction", "error in"=w279) -> ()  [unwired: 8 in, 3 out]
                n135 = local write "CurrentCmd"(w296) -> ()
                n136 = global read "Main Glb.vi" "Input Registers0-99"() -> (w285:u16[])
                n137 = call "befor_ChkSum.vi"("ToolString Input"=w296) -> ("Array"=w314:string[])  [unwired: 9 in, 1 out]
                n138 = call "Red PLC InReg.vi"("error in (no error)"=w279, "length"=10, "index"=40, "Input Registers Arr"=w285) -> ("Rad In Reg"=w281:string)  [unwired: 6 in, 1 out]
                n139 = call "Check Sum Test_01.vi"("Array"=w314) -> ("ToolStringOut_01"=w311:string, "x = y?"=w313:bool)  [unwired: 8 in, 1 out]
                "ToolStringOut_P1" <- w311
                n140 = call "Cub Meaasure FGV.vi"("Action"=Table_Save."REad" ("Enum"), "Save Index"=MeasureDisplayTab."Tray Barcode", "SN"=w281) -> ("Read Index Data"=w280:string)  [unwired: 9 in, 7 out]
                n141 = String Length(string=w311) -> (length=w309:i32)
                n142 = Not(x=w313) -> (.not. x?=w312:bool)
                n143 = global write "Main Glb.vi" "S4 Barcode ID"(w281) -> ()
                n144 = global write "Main Glb.vi" "S4 Tary ID"(w280) -> ()
                n145 = Not Equal To 0?(x=w309) -> (x != 0?=w308:bool)
                n146 = Not(x=w308) -> (.not. x?=w310:bool)
                n147 = Or(x=w312, y=w310) -> ()  [unwired: 1 out]
                n148 = call "ToolProgramTest.vi"("error in (no error)"=w294, "VISA resource name"=w297) -> ("error out"=w295:errorcluster, "Array"=w307:string[])  [unwired: 4 in, 4 out]
                "P1 Receive" <- w307
                n149 = Index Array(array=w307, index=0) -> (element=w305:string)
                n150 = Merge Errors(w295, w294) -> (w293:errorcluster)
                n151 = call "befor_ChkSum.vi"("ToolString Input"=w305) -> ("Array"=w304:string[])  [unwired: 9 in, 1 out]
                n152 = call "Check Sum Test_01.vi"("Array"=w304) -> ("ToolStringOut_01"=w300:string, "x = y?"=w301:bool)  [unwired: 8 in, 1 out]
                "ToolStringOut_P1_2" <- w300
                n153 = Unbundle By Name(w293) -> ("status"=w292:bool)
                n154 = String Length(string=w300) -> (length=w302:i32)
                n155 = Not(x=w301) -> (.not. x?=w299:bool)
                n156 = call "Get ProgReturn Info.vi"("String"=w300) -> ("Chk OK or Fail"=w287:bool)  [unwired: 8 in, 2 out]
                n157 = Not Equal To 0?(x=w302) -> (x != 0?=w303:bool)
                n158 = Not(x=w303) -> (.not. x?=w298:bool)
                n159 = Compound Arithmetic op=OR(invert w287, w299, w298) -> (w291:bool)
                n160 = Compound Arithmetic op=OR(w291, w292) -> (w290:bool)
                n161 = Increment(x=w322) -> (x+1=w331:i32)
                n162 = Not(x=w290) -> (.not. x?=w288:bool)
                n163 = Select(t=w331, s=w290, f=w322) -> (s? t:f=w328:i32)
                n164 = Greater Or Equal?(x=w328, y=w330) -> (x >= y?=w329:bool)
                n165 = case shown="True" w329 {
                  tunnel: [errorcluster {"status"=FALSE, "code"=0, "source"=""} ("error constant") errorcluster {"status"=TRUE, "code"=18402, "source"=""} ("error constant")] -> w289
                  tunnel: w328 -> [w378 _]
                  tunnel: [w378 0] -> w321
                  frame False {
                  }
                  frame True {
                  }
                }
                n166 = Increment(x=w324) -> (x+1=w332:i32)
                n167 = Select(t=w332, s=w288, f=w324) -> (s? t:f=w320:i32)
                n168 = case shown="Error .." w289 {
                  tunnel: w288 -> [w335 _]
                  tunnel: w287 -> [w334 w358]
                  frame No Error {
                    n169 = case shown="True" w335 {
                      tunnel: w334 -> [_ w336]
                      frame False {
                      }
                      frame True {
                        w355 = T13[] [enum."S4 燒入 此站不執行_46", enum."S4 燒入程式 OK_47"] items=["S2站PC動作中_20", "電流量測完成產品OK_21", "電流量測完成產品NG_22", "S2站Format 執行_23", "S2 Format OK_24", "S2 Format NG_25", "S2站燒入執行_26", "S2站燒入OK_27", "S2站燒入NG_28", "S2站動作完成_29", "S3 PC動作中_30", "S3 Format 此站執行_31", "S3 Format OK_32", "S3 Format NG_33", "S3 燒入程式 此站執行_34", "S3 燒入程式 OK_35", "S3 燒入程式 NG_36", "S3 備用_37", "S3 備用_38", "S3 動作完成_39", "S4 PC動作中_40", "S4 量測完成 產品正常_41", "S4 量測完成 產品NG_42", "S4 Format 此站執行_43", "S4 Format OK_44", "S4 Format NG_45", "S4 燒入 此站不執行_46", "S4 燒入程式 OK_47", "S4 燒入程式 NG_48", "S4 藍芽Scan OK_49", "S4 藍芽Scan NG_50", "S4 動作完成_51", "給PLC要量電流訊號", "給PLC要量電壓訊號"]
                        # "收尋S2站條碼"
                        n170 = Select(t="OK" ("DataIn"), s=w336, f="NG" ("DataIn")) -> (s? t:f=w345:string)
                        n171 = global read "Main Glb.vi" "Input Registers0-99"() -> (w338:u16[])
                        n172 = call "Auto Inspection_Status.vi"("Action"=enum16{"Initial", "Write", "Read"}."Write", "DataIn"="PROGRAM1成功", "Station"=Auto_Inspection_Station_Name2."S4Measure", "Data"=Auto_Inspection_Data_Name."ItemSN(TimeCode)") -> ()  [unwired: 9 in, 3 out]
                        n173 = call "Set OutputPLC.vi"("Address In"=20, "Array 2"=w355, "Sat Coils"=bool[] [TRUE]) -> ()  [unwired: 7 in, 1 out]
                        n174 = global read "Process Global.vi" "S4Tool Action"() -> (w353:bool[])
                        n175 = call "Red PLC InReg.vi"("length"=10, "index"=40, "Input Registers Arr"=w338) -> ("Rad In Reg"=w339:string)  [unwired: 7 in, 1 out]
                        n176 = Replace Array Subset(array=w353, new element=TRUE ("new element/subarray"), index=3) -> (w346:bool[])
                        n177 = global write "Process Global.vi" "S4Tool Action"(w346) -> ()
                        n178 = call "Cub Meaasure FGV.vi"("Action"=Table_Save."Write" ("Enum"), "Save Index"=MeasureDisplayTab."Programe(Tool Programe)", "DataIn"=w345, "SN"=w339) -> ()  [unwired: 8 in, 8 out]
                      }
                    }
                  }
                  frame Error {
                    w377 = T13[] [enum."S4 燒入 此站不執行_46", enum."S4 燒入程式 NG_48"] items=["S2站PC動作中_20", "電流量測完成產品OK_21", "電流量測完成產品NG_22", "S2站Format 執行_23", "S2 Format OK_24", "S2 Format NG_25", "S2站燒入執行_26", "S2站燒入OK_27", "S2站燒入NG_28", "S2站動作完成_29", "S3 PC動作中_30", "S3 Format 此站執行_31", "S3 Format OK_32", "S3 Format NG_33", "S3 燒入程式 此站執行_34", "S3 燒入程式 OK_35", "S3 燒入程式 NG_36", "S3 備用_37", "S3 備用_38", "S3 動作完成_39", "S4 PC動作中_40", "S4 量測完成 產品正常_41", "S4 量測完成 產品NG_42", "S4 Format 此站執行_43", "S4 Format OK_44", "S4 Format NG_45", "S4 燒入 此站不執行_46", "S4 燒入程式 OK_47", "S4 燒入程式 NG_48", "S4 藍芽Scan OK_49", "S4 藍芽Scan NG_50", "S4 動作完成_51", "給PLC要量電流訊號", "給PLC要量電壓訊號"]
                    # "收尋S2站條碼"
                    n179 = Select(t="OK" ("DataIn"), s=w358, f="NG" ("DataIn")) -> (s? t:f=w367:string)
                    n180 = global read "Main Glb.vi" "Input Registers0-99"() -> (w360:u16[])
                    n181 = call "Auto Inspection_Status.vi"("Action"=enum16{"Initial", "Write", "Read"}."Write", "DataIn"="PROGRAM1成功", "Station"=Auto_Inspection_Station_Name2."S4Measure", "Data"=Auto_Inspection_Data_Name."ItemSN(TimeCode)") -> ()  [unwired: 9 in, 3 out]
                    n182 = call "Set OutputPLC.vi"("Address In"=20, "Array 2"=w377, "Sat Coils"=bool[] [TRUE]) -> ()  [unwired: 7 in, 1 out]
                    n183 = global read "Process Global.vi" "S4Tool Action"() -> (w375:bool[])
                    n184 = call "Red PLC InReg.vi"("length"=10, "index"=40, "Input Registers Arr"=w360) -> ("Rad In Reg"=w361:string)  [unwired: 7 in, 1 out]
                    n185 = call "Cub Meaasure FGV.vi"("Action"=Table_Save."Write" ("Enum"), "Save Index"=MeasureDisplayTab."Programe(Tool Programe)", "DataIn"=w367, "SN"=w361) -> ()  [unwired: 8 in, 8 out]
                    n186 = Replace Array Subset(array=w375, new element=TRUE ("new element/subarray"), index=3) -> (w368:bool[])
                    n187 = global write "Process Global.vi" "S4Tool Action"(w368) -> ()
                  }
                }
              }
              frame "P2" {
                n188 = Increment(x=w386) -> (x+1=w385:i32)
              }
              frame "S1" {
                # "收尋S4站條碼"
                n189 = case shown="No Error" w400 {
                  frame No Error {
                    n190 = global write "Process Global.vi" "S4 Tool String Display"("S4 SCAN 等待Tool回傳") -> ()
                  }
                  frame Error {
                  }
                }
                n191 = call "Retry Num.vi"("String"=w431) -> ("Numeric"=w438:i32, "retry次數"=w435:string[])  [unwired: 9 in]
                n192 = Index Array(array=w430, index=StationCmdSelect."Command") -> (element=w427:string)
                n193 = local write "retry次數"(w435) -> ()
                n194 = call "Tool RS232 test for S4.vi"("error in (no error)"=w400, "Cmd In"=w427, "VISA resource name"=w419) -> ("error out"=w441:errorcluster, "receive string"=w390:string)  [unwired: 7 in]
                n195 = local write "CurrentCmd"(w427) -> ()
                n196 = local write "Retry"(w438) -> ()
                n197 = Unbundle By Name(w441) -> ("status"=w425:bool)
                n198 = call "befor_ChkSum.vi"("ToolString Input"=w390) -> ("ToolString Output"=w389:string)  [unwired: 9 in, 1 out]
                n199 = call "Get Scan Info for Tool.vi"("String Input"=w389) -> ("版本"=w387:string)  [unwired: 8 in, 6 out]
                n200 = call "ToolScanTest.vi"("error in (no error)"=w400, "VISA resource name"=refnum<visa-resource-name> "COM10") -> ("error out"=w407:errorcluster, "read string 6"=w413:string, "Array"=w414:string[])  [unwired: 4 in, 3 out]
                "Blue Scan receive" <- w413
                "Array" <- w414
                n201 = call "Auto Inspection_Status.vi"("Action"=enum16{"Initial", "Write", "Read"}."Write", "DataIn"="SCAN1", "Station"=Auto_Inspection_Station_Name2."S4Measure", "Data"=Auto_Inspection_Data_Name."CurrentAction", "error in"=w400) -> ("error out"=w391:errorcluster)  [unwired: 8 in, 2 out]
                n202 = global read "Main Glb.vi" "Input Registers0-99"() -> (w396:u16[])
                n203 = String Length(string=w413) -> (length=w412:i32)
                n204 = Not Equal?(x=w412, y=0) -> (x != y?=w410:bool)
                n205 = call <vilib>:"Clear Errors.vi"("error in (no error)"=w407) -> ()  [unwired: 5 in, 2 out]
                n206 = call "Check Sum Test_01.vi"("Array"=w414) -> ("ToolStringOut_01"=w401:string, "ChkSum"=→"S1 ChkSum":string, "x = y?"=w416:bool)  [unwired: 8 in]
                "S1 ToolStringOut" <- w401
                n207 = Not(x=w410) -> (.not. x?=w409:bool)
                n208 = call "Red PLC InReg.vi"("error in (no error)"=w391, "length"=10, "index"=40, "Input Registers Arr"=w396) -> ("Rad In Reg"=w388:string)  [unwired: 6 in, 1 out]
                n209 = disable-structure shown="Disabled" {
                  disable-tunnel: w388 -> [w443 _]
                  disable-tunnel: w387 -> [w442 _]
                  frame Disabled {
                    n210 = call "Cub Meaasure PD FGV.vi"("Action"=Table_Save."Write", "Save low Index"=PD_Table_Save_Low_Index."low 3", "Save Col Index"=PD_Table_Save_Col_Index."433半成品 版本_H", "DataIn"=w442, "SN"=w443) -> ()  [unwired: 7 in, 8 out]
                  }
                  frame Enabled {
                  }
                }
                n211 = global write "Process Global.vi" "S4 Tool String Display"(w401) -> ()
                n212 = call "Cub Meaasure FGV.vi"("Action"=Table_Save."REad" ("Enum"), "Save Index"=MeasureDisplayTab."Tray Barcode", "SN"=w388) -> ("Read Index Data"=w392:string)  [unwired: 9 in, 7 out]
                n213 = Not(x=w416) -> (.not. x?=w406:bool)
                n214 = Or(x=w406, y=w409) -> (x .or. y?=w404:bool)
                n215 = global write "Main Glb.vi" "S4 Barcode ID"(w388) -> ()
                n216 = global write "Main Glb.vi" "S4 Tary ID"(w392) -> ()
                n217 = Not(x=w404) -> (.not. x?=w403:bool)
                n218 = Or(x=w404, y=w425) -> (x .or. y?=w424:bool)
                n219 = call "Scan Data Save.vi"("error in (no error)"=w407, "index"=40, "OK and NG"=w403, "String In"=w401) -> ("error out"=w405:errorcluster)  [unwired: 7 in]
                n220 = Not(x=w424) -> (.not. x?=w398:bool)
                n221 = Increment(x=w428) -> (x+1=w439:i32)
                n222 = Increment(x=w429) -> (x+1=w440:i32)
                n223 = Select(t=w439, s=w424, f=w428) -> (s? t:f=w436:i32)
                n224 = Greater Or Equal?(x=w436, y=w438) -> (x >= y?=w437:bool)
                n225 = case shown="False" w398 {
                  frame False {
                    n226 = call "Auto Inspection_Status.vi"("Action"=enum16{"Initial", "Write", "Read"}."Write", "DataIn"="SCAN1 RETRY", "Station"=Auto_Inspection_Station_Name2."S4Measure", "Data"=Auto_Inspection_Data_Name."ItemSN(TimeCode)") -> ()  [unwired: 9 in, 3 out]
                  }
                  frame True {
                  }
                }
                n227 = Select(t=w440, s=w398, f=w429) -> (s? t:f=w433:i32)
                n228 = case shown="False" w437 {
                  tunnel: [errorcluster {"status"=FALSE, "code"=0, "source"=""} ("error constant") errorcluster {"status"=TRUE, "code"=18403, "source"=""} ("error constant")] -> w399
                  tunnel: w436 -> [w482 _]
                  tunnel: [w482 0] -> w432
                  frame False {
                  }
                  frame True {
                  }
                }
                n229 = case shown="Error .." w399 {
                  tunnel: [w453 w472] -> w408
                  tunnel: w398 -> [w452 _]
                  frame No Error {
                    n230 = case shown="True" w452 {
                      tunnel: [_ w459] -> w453
                      frame False {
                      }
                      frame True {
                        w466 = T13[] [enum."S4 藍芽Scan OK_49"] items=["S2站PC動作中_20", "電流量測完成產品OK_21", "電流量測完成產品NG_22", "S2站Format 執行_23", "S2 Format OK_24", "S2 Format NG_25", "S2站燒入執行_26", "S2站燒入OK_27", "S2站燒入NG_28", "S2站動作完成_29", "S3 PC動作中_30", "S3 Format 此站執行_31", "S3 Format OK_32", "S3 Format NG_33", "S3 燒入程式 此站執行_34", "S3 燒入程式 OK_35", "S3 燒入程式 NG_36", "S3 備用_37", "S3 備用_38", "S3 動作完成_39", "S4 PC動作中_40", "S4 量測完成 產品正常_41", "S4 量測完成 產品NG_42", "S4 Format 此站執行_43", "S4 Format OK_44", "S4 Format NG_45", "S4 燒入 此站不執行_46", "S4 燒入程式 OK_47", "S4 燒入程式 NG_48", "S4 藍芽Scan OK_49", "S4 藍芽Scan NG_50", "S4 動作完成_51", "給PLC要量電流訊號", "給PLC要量電壓訊號"]
                        n231 = global read "Process Global.vi" "S4Tool Action"() -> (w458:bool[])
                        n232 = Replace Array Subset(array=w458, new element=TRUE ("new element/subarray"), index=4) -> (w455:bool[])
                        n233 = global write "Process Global.vi" "S4Tool Action"(w455) -> ()
                        n234 = call "Set OutputPLC.vi"("Address In"=20, "Array 2"=w466, "Sat Coils"=bool[] [TRUE]) -> ("Error Out"=w461:errorcluster[])  [unwired: 7 in]
                        n235 = Merge Errors(w461) -> (w460:errorcluster)
                        n236 = call "Auto Inspection_Status.vi"("Action"=enum16{"Initial", "Write", "Read"}."Write", "DataIn"="SCAN1 成功", "Station"=Auto_Inspection_Station_Name2."S4Measure", "Data"=Auto_Inspection_Data_Name."ItemSN(TimeCode)", "error in"=w460) -> ("error out"=w459:errorcluster)  [unwired: 8 in, 2 out]
                      }
                    }
                  }
                  frame Error {
                    w481 = T13[] [enum."S4 藍芽Scan NG_50"] items=["S2站PC動作中_20", "電流量測完成產品OK_21", "電流量測完成產品NG_22", "S2站Format 執行_23", "S2 Format OK_24", "S2 Format NG_25", "S2站燒入執行_26", "S2站燒入OK_27", "S2站燒入NG_28", "S2站動作完成_29", "S3 PC動作中_30", "S3 Format 此站執行_31", "S3 Format OK_32", "S3 Format NG_33", "S3 燒入程式 此站執行_34", "S3 燒入程式 OK_35", "S3 燒入程式 NG_36", "S3 備用_37", "S3 備用_38", "S3 動作完成_39", "S4 PC動作中_40", "S4 量測完成 產品正常_41", "S4 量測完成 產品NG_42", "S4 Format 此站執行_43", "S4 Format OK_44", "S4 Format NG_45", "S4 燒入 此站不執行_46", "S4 燒入程式 OK_47", "S4 燒入程式 NG_48", "S4 藍芽Scan OK_49", "S4 藍芽Scan NG_50", "S4 動作完成_51", "給PLC要量電流訊號", "給PLC要量電壓訊號"]
                    n237 = global read "Process Global.vi" "S4Tool Action"() -> (w471:bool[])
                    n238 = Replace Array Subset(array=w471, new element=FALSE ("new element/subarray"), index=4) -> (w468:bool[])
                    n239 = call "Set OutputPLC.vi"("Address In"=20, "Array 2"=w481, "Sat Coils"=bool[] [TRUE]) -> ("Error Out"=w474:errorcluster[])  [unwired: 7 in]
                    n240 = global write "Process Global.vi" "S4Tool Action"(w468) -> ()
                    n241 = Merge Errors(w474) -> (w473:errorcluster)
                    n242 = call "Auto Inspection_Status.vi"("Action"=enum16{"Initial", "Write", "Read"}."Write", "DataIn"="SCAN1 失敗", "Station"=Auto_Inspection_Station_Name2."S4Measure", "Data"=Auto_Inspection_Data_Name."ItemSN(TimeCode)", "error in"=w473) -> ("error out"=w472:errorcluster)  [unwired: 8 in, 2 out]
                  }
                }
                n243 = Merge Errors(w405, w408, w399) -> (w418:errorcluster)
              }
              frame "S2" {
                # "收尋S4站條碼"
                # "要在一個S2的 SAVE"
                # "收尋S4站條碼"
                n244 = global read "Main Glb.vi" "Input Registers0-99"() -> (w492:u16[])
                n245 = call "Red PLC InReg.vi"("error in (no error)"=w486, "length"=10, "index"=40, "Input Registers Arr"=w492) -> ("Rad In Reg"=w488:string)  [unwired: 6 in, 1 out]
                n246 = call "Auto Inspection_Status.vi"("Action"=enum16{"Initial", "Write", "Read"}."Write", "DataIn"="SCAN2", "Station"=Auto_Inspection_Station_Name2."S4Measure", "Data"=Auto_Inspection_Data_Name."CurrentAction", "error in"=w486) -> ()  [unwired: 8 in, 3 out]
                n247 = call "Cub Meaasure FGV.vi"("Action"=Table_Save."REad" ("Enum"), "Save Index"=MeasureDisplayTab."Tray Barcode", "SN"=w488) -> ("Read Index Data"=w487:string)  [unwired: 9 in, 7 out]
                n248 = global write "Main Glb.vi" "S4 Barcode ID"(w488) -> ()
                n249 = global write "Main Glb.vi" "S4 Tary ID"(w487) -> ()
                n250 = call "Retry Num.vi"("String"=w535) -> ("Numeric"=w525:i32, "retry次數"=w522:string[])  [unwired: 9 in]
                n251 = Index Array(array=w536, index=StationCmdSelect."Command") -> (element=w521:string)
                n252 = call "ToolScanTest.vi"("error in (no error)"=w486, "VISA resource name"=refnum<visa-resource-name> "COM10") -> ("error out"=w520:errorcluster, "read string 3"=w518:string)  [unwired: 4 in, 4 out]
                "Blue Scan2 receive" <- w518
                n253 = local write "retry次數"(w522) -> ()
                n254 = call "Tool RS232 test for S4.vi"("error in (no error)"=w486, "Cmd In"=w521, "VISA resource name"=w530) -> ("error out"=w528:errorcluster, "receive string"=→"S2 receive":string)  [unwired: 7 in]
                n255 = local write "CurrentCmd"(w521) -> ()
                n256 = call <vilib>:"Clear Errors.vi"("error in (no error)"=w520) -> ()  [unwired: 5 in, 2 out]
                n257 = local write "Retry"(w525) -> ()
                n258 = Unbundle By Name(w528) -> ("status"=w515:bool)
                n259 = String Length(string=w518) -> (length=w519:i32)
                n260 = Not Equal To 0?(x=w519) -> (x != 0?=w517:bool)
                n261 = Not(x=w517) -> (.not. x?=w516:bool)
                n262 = Or(x=w516, y=w515) -> (x .or. y?=w514:bool)
                n263 = Not(x=w514) -> (.not. x?=w494:bool)
                n264 = Increment(x=w534) -> (x+1=w526:i32)
                n265 = Select(t=w526, s=w514, f=w534) -> (s? t:f=w523:i32)
                n266 = Greater Or Equal?(x=w523, y=w525) -> (x >= y?=w524:bool)
                n267 = case shown="False" w494 {
                  frame False {
                    n268 = call "Auto Inspection_Status.vi"("Action"=enum16{"Initial", "Write", "Read"}."Write", "DataIn"="SCAN2 RETRY", "Station"=Auto_Inspection_Station_Name2."S4Measure", "Data"=Auto_Inspection_Data_Name."ItemSN(TimeCode)") -> ()  [unwired: 9 in, 3 out]
                  }
                  frame True {
                  }
                }
                n269 = case shown="True" w524 {
                  tunnel: [errorcluster {"status"=FALSE, "code"=0, "source"=""} ("error constant") errorcluster {"status"=TRUE, "code"=18404, "source"=""} ("error constant")] -> w499
                  tunnel: w523 -> [w569 _]
                  tunnel: [w569 0] -> w532
                  frame False {
                  }
                  frame True {
                  }
                }
                n270 = Increment(x=w537) -> (x+1=w527:i32)
                n271 = Select(t=w527, s=w494, f=w537) -> (s? t:f=w533:i32)
                n272 = Unbundle By Name(w499) -> ("status"=w501:bool)
                n273 = Not(x=w501) -> (.not. x?=w500:bool)
                n274 = case shown="Error .." w499 {
                  tunnel: [w544 w566] -> w511
                  tunnel: w494 -> [w543 _]
                  frame No Error {
                    n275 = case shown="True" w543 {
                      tunnel: [_ w555] -> w544
                      frame False {
                      }
                      frame True {
                        w554 = T13[] [enum."S4 藍芽Scan OK_49"] items=["S2站PC動作中_20", "電流量測完成產品OK_21", "電流量測完成產品NG_22", "S2站Format 執行_23", "S2 Format OK_24", "S2 Format NG_25", "S2站燒入執行_26", "S2站燒入OK_27", "S2站燒入NG_28", "S2站動作完成_29", "S3 PC動作中_30", "S3 Format 此站執行_31", "S3 Format OK_32", "S3 Format NG_33", "S3 燒入程式 此站執行_34", "S3 燒入程式 OK_35", "S3 燒入程式 NG_36", "S3 備用_37", "S3 備用_38", "S3 動作完成_39", "S4 PC動作中_40", "S4 量測完成 產品正常_41", "S4 量測完成 產品NG_42", "S4 Format 此站執行_43", "S4 Format OK_44", "S4 Format NG_45", "S4 燒入 此站不執行_46", "S4 燒入程式 OK_47", "S4 燒入程式 NG_48", "S4 藍芽Scan OK_49", "S4 藍芽Scan NG_50", "S4 動作完成_51", "給PLC要量電流訊號", "給PLC要量電壓訊號"]
                        n276 = call "Auto Inspection_Status.vi"("Action"=enum16{"Initial", "Write", "Read"}."Write", "DataIn"="SCAN2 成功", "Station"=Auto_Inspection_Station_Name2."S4Measure", "Data"=Auto_Inspection_Data_Name."ItemSN(TimeCode)") -> ()  [unwired: 9 in, 3 out]
                        n277 = global read "Process Global.vi" "S4Tool Action"() -> (w553:bool[])
                        n278 = call "Set OutputPLC.vi"("Address In"=20, "Array 2"=w554, "Sat Coils"=bool[] [TRUE]) -> ("Error Out"=w555:errorcluster[])  [unwired: 7 in]
                        n279 = Replace Array Subset(array=w553, new element=TRUE ("new element/subarray"), index=4) -> (w546:bool[])
                        n280 = global write "Process Global.vi" "S4Tool Action"(w546) -> ()
                      }
                    }
                  }
                  frame Error {
                    w568 = T13[] [enum."S4 藍芽Scan NG_50"] items=["S2站PC動作中_20", "電流量測完成產品OK_21", "電流量測完成產品NG_22", "S2站Format 執行_23", "S2 Format OK_24", "S2 Format NG_25", "S2站燒入執行_26", "S2站燒入OK_27", "S2站燒入NG_28", "S2站動作完成_29", "S3 PC動作中_30", "S3 Format 此站執行_31", "S3 Format OK_32", "S3 Format NG_33", "S3 燒入程式 此站執行_34", "S3 燒入程式 OK_35", "S3 燒入程式 NG_36", "S3 備用_37", "S3 備用_38", "S3 動作完成_39", "S4 PC動作中_40", "S4 量測完成 產品正常_41", "S4 量測完成 產品NG_42", "S4 Format 此站執行_43", "S4 Format OK_44", "S4 Format NG_45", "S4 燒入 此站不執行_46", "S4 燒入程式 OK_47", "S4 燒入程式 NG_48", "S4 藍芽Scan OK_49", "S4 藍芽Scan NG_50", "S4 動作完成_51", "給PLC要量電流訊號", "給PLC要量電壓訊號"]
                    n281 = global read "Process Global.vi" "S4Tool Action"() -> (w564:bool[])
                    n282 = call "Auto Inspection_Status.vi"("Action"=enum16{"Initial", "Write", "Read"}."Write", "DataIn"="SCAN2 失敗", "Station"=Auto_Inspection_Station_Name2."S4Measure", "Data"=Auto_Inspection_Data_Name."ItemSN(TimeCode)") -> ()  [unwired: 9 in, 3 out]
                    n283 = call "Set OutputPLC.vi"("Address In"=20, "Array 2"=w568, "Sat Coils"=bool[] [TRUE]) -> ("Error Out"=w566:errorcluster[])  [unwired: 7 in]
                    n284 = Replace Array Subset(array=w564, new element=FALSE ("new element/subarray"), index=4) -> (w557:bool[])
                    n285 = global write "Process Global.vi" "S4Tool Action"(w557) -> ()
                  }
                }
                n286 = Select(t="OK" ("DataIn"), s=w500, f="NG" ("DataIn")) -> (s? t:f=w510:string)
                n287 = global read "Main Glb.vi" "Input Registers0-99"() -> (w503:u16[])
                n288 = Merge Errors(w511, w499) -> (w531:errorcluster)
                n289 = call "Red PLC InReg.vi"("length"=10, "index"=40, "Input Registers Arr"=w503) -> ("Rad In Reg"=w504:string)  [unwired: 7 in, 1 out]
                n290 = call "Cub Meaasure FGV.vi"("Action"=Table_Save."Write" ("Enum"), "Save Index"=MeasureDisplayTab."ASKscan_433(ASK scan)", "DataIn"=w510, "SN"=w504) -> ()  [unwired: 8 in, 8 out]
              }
              frame "D" {
                n291 = Index Array(array=w584) -> (element=w583:i32)  [unwired: 1 in]
                n292 = Multiply(x=1000, y=w583) -> (x*y=w582:i32)
                n293 = Wait (ms)(milliseconds to wait=w582) -> ()  [unwired: 1 out]
                n294 = call "Auto Inspection_Status.vi"("Action"=enum16{"Initial", "Write", "Read"}."Write", "DataIn"="Delay Time", "Station"=Auto_Inspection_Station_Name2."S4Measure", "Data"=Auto_Inspection_Data_Name."CurrentAction") -> ()  [unwired: 9 in, 3 out]
                n295 = Increment(x=w579) -> (x+1=w578:i32)
              }
              frame "T1" {
                w592 = T13[] [enum."給PLC要量電流訊號"] items=["S2站PC動作中_20", "電流量測完成產品OK_21", "電流量測完成產品NG_22", "S2站Format 執行_23", "S2 Format OK_24", "S2 Format NG_25", "S2站燒入執行_26", "S2站燒入OK_27", "S2站燒入NG_28", "S2站動作完成_29", "S3 PC動作中_30", "S3 Format 此站執行_31", "S3 Format OK_32", "S3 Format NG_33", "S3 燒入程式 此站執行_34", "S3 燒入程式 OK_35", "S3 燒入程式 NG_36", "S3 備用_37", "S3 備用_38", "S3 動作完成_39", "S4 PC動作中_40", "S4 量測完成 產品正常_41", "S4 量測完成 產品NG_42", "S4 Format 此站執行_43", "S4 Format OK_44", "S4 Format NG_45", "S4 燒入 此站不執行_46", "S4 燒入程式 OK_47", "S4 燒入程式 NG_48", "S4 藍芽Scan OK_49", "S4 藍芽Scan NG_50", "S4 動作完成_51", "給PLC要量電流訊號", "給PLC要量電壓訊號"]
                n296 = flat-sequence {
                  tunnel: [w601] -> w590
                  tunnel: w593 -> [_]
                  frame #0 {
                    n297 = global read "Main Glb.vi" "Discrete Inputs"() -> (w603:bool[])
                    n298 = Index Array(array=w603, index=S2_Station_Input."21_PLC下達可測電流訊號" ("Enum")) -> (element=w601:bool)
                  }
                }
                n299 = call "ModbusCmdIn.vi"("data"=T9 {"starting address"=0, "number of inputs"=0, "Sat Coils"=[], "Holding Registers"=[]}, "Enum"=ModbusCmd."Fetch Discrete Inputs") -> ("error out"=w586:errorcluster)  [unwired: 9 in]
                n300 = call "Set OutputPLC.vi"("Address In"=20, "Array 2"=w592, "Sat Coils"=bool[] [TRUE], "error in (no error)"=w586) -> ("Error Out"=w593:errorcluster[])  [unwired: 6 in]
                n301 = case shown="True" w590 {
                  tunnel: w599 -> [_ w644]
                  tunnel: w598 -> [_ w643]
                  tunnel: [0 ("Err Count") w641] -> w597
                  tunnel: w596 -> [w607 w640]
                  tunnel: [w607 w638] -> w595
                  tunnel: [errorcluster {"status"=FALSE, "code"=0, "source"=""} ("error IO") w618] -> w594
                  frame False {
                    n302 = Wait (ms)(milliseconds to wait=u32 250) -> ()  [unwired: 1 out]
                  }
                  frame True {
                    w648 = u16 3 items=["SYSTem:VERSion?", "SYSTem:ERRor?", "*IDN?", "MEAS:CURR:DC?", "MEAS:VOLT?", "SYSTem:ERRor?"] ("Ringfor34450A")
                    w647 = u16 5 items=["SYSTem:VERSion?", "SYSTem:ERRor?", "*IDN?", "MEAS:CURR:DC?", "MEAS:VOLT?", "MEAS:VOLT:DC?"] ("RingforIT8511")
                    w645 = u16 1 items=["IT8511", "34450A", "WRBuff"] ("ChangeStatus")
                    # "收尋S2站條碼"
                    # "T1 34450A/"
                    # "量電流"
                    n303 = call "Retry Num.vi"("String"=w643) -> ("Numeric"=w650:i32, "retry次數"=w649:string[])  [unwired: 9 in]
                    n304 = call "Auto Inspection_Status.vi"("Action"=enum16{"Initial", "Write", "Read"}."Write", "DataIn"="儀器測量", "Station"=Auto_Inspection_Station_Name2."S4Measure", "Data"=Auto_Inspection_Data_Name."CurrentAction") -> ()  [unwired: 9 in, 3 out]
                    n305 = local write "retry次數"(w649) -> ()
                    n306 = local write "Retry"(w650) -> ()
                    n307 = call "MTool34450A.vi"("Ringfor34450A"=w648, "RingforIT8511"=w647, "VISA resource name"=refnum<visa-resource-name> "USB0::0x2A8D::0xB318::MY59430005::INSTR", "ChangeStatus"=w645) -> ("error out"=w636:errorcluster, 1:"μA"=w616:string, 2:"μA"=w611:dbl, "read buffer"=w633:string)  [unwired: 4 in]
                    "T1 buffer" <- w633
                    n308 = call "ProjectSearchDataName.vi"("element"="$ForceSetBinChk_") -> ("variant"=w613:variant)  [unwired: 7 in, 3 out]
                    n309 = Variant To Data(type=FALSE, Variant=w613) -> (data=w612:bool)  [unwired: 1 in, 1 out]
                    n310 = call "NG Pack量測值轉換.vi"("位數"=4, "input string"=w633, "PLC address"=20) -> ("error out"=w627:errorcluster)  [unwired: 7 in, 1 out]
                    n311 = Unbundle By Name(w636) -> ("status"=w639:bool)
                    n312 = Increment(x=w644) -> (x+1=w651:i32)
                    n313 = global write "Process Global.vi" "T1 Current00"(w611) -> ()
                    n314 = Select(t=w651, s=w639, f=w644) -> (s? t:f=w642:i32)
                    n315 = Greater Or Equal?(x=w642, y=w650) -> (x >= y?=w637:bool)
                    n316 = Not(x=w639) -> (.not. x?=w610:bool)
                    n317 = case shown="True" w612 {
                      tunnel: w611 -> [w655 w660]
                      tunnel: [w656 w659] -> w609
                      tunnel: w610 -> [w656 _]
                      frame False {
                        n318 = Number To Fractional String(number=w655) -> (F-format string=w653:string)  [unwired: 3 in]
                        n319 = String Subset(string=w653, length (rest)=5 ("length (rest)")) -> ()  [unwired: 1 in, 1 out]
                      }
                      frame True {
                        n320 = call "ProjectSearchDataName.vi"("element"="$Current Up") -> ("variant"=w665:variant)  [unwired: 7 in, 3 out]
                        n321 = call "ProjectSearchDataName.vi"("element"="$Current Dn") -> ("variant"=w664:variant)  [unwired: 7 in, 3 out]
                        n322 = Variant To Data(type=0.0, Variant=w665) -> (data=w662:dbl)  [unwired: 1 in, 1 out]
                        n323 = Variant To Data(type=0.0, Variant=w664) -> (data=w661:dbl)  [unwired: 1 in, 1 out]
                        n324 = In Range and Coerce(upper limit=w662, x=w660, lower limit=w661) -> (In Range?=w659:bool)  [unwired: 1 out]
                      }
                    }
                    n325 = case shown="True" w637 {
                      tunnel: [errorcluster {"status"=FALSE, "code"=0, "source"=""} ("error constant") errorcluster {"status"=TRUE, "code"=18405, "source"=""} ("error constant")] -> w632
                      tunnel: w642 -> [w690 _]
                      tunnel: [w690 0] -> w641
                      tunnel: w636 -> [_ _]
                      frame False {
                      }
                      frame True {
                      }
                    }
                    n326 = Increment(x=w640) -> (x+1=w652:i32)
                    n327 = Select(t=w652, s=w609, f=w640) -> (s? t:f=w638:i32)
                    n328 = Merge Errors(w627, w632) -> (w608:errorcluster)
                    n329 = global read "Main Glb.vi" "Input Registers0-99"() -> (w620:u16[])
                    n330 = Select(t=w616, s=w609, f="NG" ("DataIn")) -> (s? t:f=w626:string)
                    n331 = case shown="Error .." w608 {
                      tunnel: [w668 w687] -> w619
                      tunnel: w609 -> [w667 _]
                      frame No Error {
                        n332 = case shown="True" w667 {
                          tunnel: [_ w673] -> w668
                          frame False {
                          }
                          frame True {
                            w677 = T13[] [enum."給PLC要量電流訊號"] items=["S2站PC動作中_20", "電流量測完成產品OK_21", "電流量測完成產品NG_22", "S2站Format 執行_23", "S2 Format OK_24", "S2 Format NG_25", "S2站燒入執行_26", "S2站燒入OK_27", "S2站燒入NG_28", "S2站動作完成_29", "S3 PC動作中_30", "S3 Format 此站執行_31", "S3 Format OK_32", "S3 Format NG_33", "S3 燒入程式 此站執行_34", "S3 燒入程式 OK_35", "S3 燒入程式 NG_36", "S3 備用_37", "S3 備用_38", "S3 動作完成_39", "S4 PC動作中_40", "S4 量測完成 產品正常_41", "S4 量測完成 產品NG_42", "S4 Format 此站執行_43", "S4 Format OK_44", "S4 Format NG_45", "S4 燒入 此站不執行_46", "S4 燒入程式 OK_47", "S4 燒入程式 NG_48", "S4 藍芽Scan OK_49", "S4 藍芽Scan NG_50", "S4 動作完成_51", "給PLC要量電流訊號", "給PLC要量電壓訊號"]
                            w680 = T13[] [enum."電流量測完成產品OK_21"] items=["S2站PC動作中_20", "電流量測完成產品OK_21", "電流量測完成產品NG_22", "S2站Format 執行_23", "S2 Format OK_24", "S2 Format NG_25", "S2站燒入執行_26", "S2站燒入OK_27", "S2站燒入NG_28", "S2站動作完成_29", "S3 PC動作中_30", "S3 Format 此站執行_31", "S3 Format OK_32", "S3 Format NG_33", "S3 燒入程式 此站執行_34", "S3 燒入程式 OK_35", "S3 燒入程式 NG_36", "S3 備用_37", "S3 備用_38", "S3 動作完成_39", "S4 PC動作中_40", "S4 量測完成 產品正常_41", "S4 量測完成 產品NG_42", "S4 Format 此站執行_43", "S4 Format OK_44", "S4 Format NG_45", "S4 燒入 此站不執行_46", "S4 燒入程式 OK_47", "S4 燒入程式 NG_48", "S4 藍芽Scan OK_49", "S4 藍芽Scan NG_50", "S4 動作完成_51", "給PLC要量電流訊號", "給PLC要量電壓訊號"]
                            n333 = global read "Process Global.vi" "S4Tool Action"() -> (w671:bool[])
                            n334 = call "Set OutputPLC.vi"("Address In"=20, "Array 2"=w680, "Sat Coils"=bool[] [TRUE]) -> ("Error Out"=w675:errorcluster[])  [unwired: 7 in]
                            n335 = Merge Errors(w675) -> (w674:errorcluster)
                            n336 = Replace Array Subset(array=w671, new element=TRUE ("new element/subarray"), index=5) -> (w672:bool[])
                            n337 = global write "Process Global.vi" "S4Tool Action"(w672) -> ()
                            n338 = call "Set OutputPLC.vi"("Address In"=20, "Array 2"=w677, "Sat Coils"=bool[] [FALSE], "error in (no error)"=w674) -> ("Error Out"=w673:errorcluster[])  [unwired: 6 in]
                          }
                        }
                      }
                      frame Error {
                        w689 = T13[] [enum."電流量測完成產品NG_22", enum."S2站PC動作中_20"] items=["S2站PC動作中_20", "電流量測完成產品OK_21", "電流量測完成產品NG_22", "S2站Format 執行_23", "S2 Format OK_24", "S2 Format NG_25", "S2站燒入執行_26", "S2站燒入OK_27", "S2站燒入NG_28", "S2站動作完成_29", "S3 PC動作中_30", "S3 Format 此站執行_31", "S3 Format OK_32", "S3 Format NG_33", "S3 燒入程式 此站執行_34", "S3 燒入程式 OK_35", "S3 燒入程式 NG_36", "S3 備用_37", "S3 備用_38", "S3 動作完成_39", "S4 PC動作中_40", "S4 量測完成 產品正常_41", "S4 量測完成 產品NG_42", "S4 Format 此站執行_43", "S4 Format OK_44", "S4 Format NG_45", "S4 燒入 此站不執行_46", "S4 燒入程式 OK_47", "S4 燒入程式 NG_48", "S4 藍芽Scan OK_49", "S4 藍芽Scan NG_50", "S4 動作完成_51", "給PLC要量電流訊號", "給PLC要量電壓訊號"]
                        n339 = call "Set OutputPLC.vi"("Address In"=20, "Array 2"=w689, "Sat Coils"=bool[] [TRUE]) -> ("Error Out"=w687:errorcluster[])  [unwired: 7 in]
                        n340 = global read "Process Global.vi" "S4Tool Action"() -> (w684:bool[])
                        n341 = Replace Array Subset(array=w684, new element=FALSE ("new element/subarray"), index=5) -> (w685:bool[])
                        n342 = global write "Process Global.vi" "S4Tool Action"(w685) -> ()
                      }
                    }
                    n343 = call "Red PLC InReg.vi"("length"=10, "index"=40, "Input Registers Arr"=w620) -> ("Rad In Reg"=w621:string)  [unwired: 7 in, 1 out]
                    n344 = call "Cub Meaasure FGV.vi"("Action"=Table_Save."Write" ("Enum"), "Save Index"=MeasureDisplayTab."耗電流 uA(電流表)", "DataIn"=w626, "SN"=w621) -> ()  [unwired: 8 in, 8 out]
                    n345 = Merge Errors(w619, w608) -> (w618:errorcluster)
                  }
                }
              }
              frame "T2" {
                w701 = T13[] [enum."給PLC要量電壓訊號"] items=["S2站PC動作中_20", "電流量測完成產品OK_21", "電流量測完成產品NG_22", "S2站Format 執行_23", "S2 Format OK_24", "S2 Format NG_25", "S2站燒入執行_26", "S2站燒入OK_27", "S2站燒入NG_28", "S2站動作完成_29", "S3 PC動作中_30", "S3 Format 此站執行_31", "S3 Format OK_32", "S3 Format NG_33", "S3 燒入程式 此站執行_34", "S3 燒入程式 OK_35", "S3 燒入程式 NG_36", "S3 備用_37", "S3 備用_38", "S3 動作完成_39", "S4 PC動作中_40", "S4 量測完成 產品正常_41", "S4 量測完成 產品NG_42", "S4 Format 此站執行_43", "S4 Format OK_44", "S4 Format NG_45", "S4 燒入 此站不執行_46", "S4 燒入程式 OK_47", "S4 燒入程式 NG_48", "S4 藍芽Scan OK_49", "S4 藍芽Scan NG_50", "S4 動作完成_51", "給PLC要量電流訊號", "給PLC要量電壓訊號"]
                n346 = flat-sequence {
                  tunnel: [w711] -> w698
                  tunnel: w702 -> [w710]
                  tunnel: [w710] -> w697
                  frame #0 {
                    n347 = global read "Main Glb.vi" "Discrete Inputs"() -> (w713:bool[])
                    n348 = Index Array(array=w713, index=S2_Station_Input."22_PLC下達可測電壓訊號" ("Enum")) -> (element=w711:bool)
                  }
                }
                n349 = call "ModbusCmdIn.vi"("data"=T9 {"starting address"=0, "number of inputs"=0, "Sat Coils"=[], "Holding Registers"=[]}, "Enum"=ModbusCmd."Fetch Discrete Inputs") -> ("error out"=w694:errorcluster)  [unwired: 9 in]
                n350 = call "Set OutputPLC.vi"("Address In"=20, "Array 2"=w701, "Sat Coils"=bool[] [TRUE], "error in (no error)"=w694) -> ("Error Out"=w702:errorcluster[])  [unwired: 6 in]
                n351 = case shown="True" w698 {
                  tunnel: [0 w752] -> w708
                  tunnel: w707 -> [w721 w751]
                  tunnel: [w721 w750] -> w706
                  tunnel: w705 -> [_ w749]
                  tunnel: w704 -> [_ w748]
                  tunnel: [errorcluster {"status"=FALSE, "code"=0, "source"=""} ("error IO") w722] -> w703
                  tunnel: w697 -> [_ _]
                  frame False {
                    n352 = call "Auto Inspection_Status.vi"("Action"=enum16{"Initial", "Write", "Read"}."Write", "DataIn"="等待PLC可量測訊號", "Station"=Auto_Inspection_Station_Name2."S4Measure", "Data"=Auto_Inspection_Data_Name."CurrentAction") -> ()  [unwired: 9 in, 3 out]
                    n353 = Wait (ms)(milliseconds to wait=250) -> ()  [unwired: 1 out]
                  }
                  frame True {
                    w756 = u16 3 items=["SYSTem:VERSion?", "SYSTem:ERRor?", "*IDN?", "MEAS:CURR:DC?", "MEAS:VOLT?", "SYSTem:ERRor?"] ("Ringfor34450A")
                    w755 = u16 5 items=["SYSTem:VERSion?", "SYSTem:ERRor?", "*IDN?", "MEAS:CURR:DC?", "MEAS:VOLT?", "MEAS:VOLT:DC?"] ("RingforIT8511")
                    w753 = u16 0 items=["IT8511", "34450A", "WRBuff"] ("ChangeStatus")
                    # "收尋S2站條碼"
                    # "量電壓"
                    # "T2  T8511A/COM11"
                    n354 = call "Retry Num.vi"("String"=w749) -> ("Numeric"=w762:i32, "retry次數"=w761:string[])  [unwired: 9 in]
                    n355 = call "Auto Inspection_Status.vi"("Action"=enum16{"Initial", "Write", "Read"}."Write", "DataIn"="儀器測量", "Station"=Auto_Inspection_Station_Name2."S4Measure", "Data"=Auto_Inspection_Data_Name."CurrentAction") -> ()  [unwired: 9 in, 3 out]
                    n356 = local write "retry次數"(w761) -> ()
                    n357 = local write "Retry"(w762) -> ()
                    n358 = call "MTool34450A.vi"("Ringfor34450A"=w756, "RingforIT8511"=w755, "VISA resource name"=refnum<visa-resource-name> "COM11", "ChangeStatus"=w753) -> ("error out"=w757:errorcluster, "read buffer"=w726:string)  [unwired: 4 in, 2 out]
                    "T2 buffer" <- w726
                    n359 = call "ProjectSearchDataName.vi"("element"="$ForceSetBinChk_") -> ("variant"=w730:variant)  [unwired: 7 in, 3 out]
                    n360 = Unbundle By Name(w757) -> ("status"=w759:bool)
                    n361 = Variant To Data(type=FALSE, Variant=w730) -> (data=w727:bool)  [unwired: 1 in, 1 out]
                    n362 = global write "Process Global.vi" "T2 Voltage"(w726) -> ()
                    n363 = Increment(x=w748) -> (x+1=w747:i32)
                    n364 = Fract/Exp String To Number(string=w726) -> (number=w725:dbl)  [unwired: 3 in, 1 out]
                    n365 = Select(t=w747, s=w759, f=w747) -> (s? t:f=w760:i32)
                    n366 = call "NG Pack量測值轉換.vi"("位數"=6, "input string"=w726, "PLC address"=40) -> ("error out"=w744:errorcluster)  [unwired: 7 in, 1 out]
                    n367 = Greater Or Equal?(x=w760, y=w762) -> (x >= y?=w758:bool)
                    n368 = case shown="True" w758 {
                      tunnel: [errorcluster {"status"=FALSE, "code"=0, "source"=""} ("error constant") errorcluster {"status"=TRUE, "code"=18406, "source"=""} ("error constant")] -> w743
                      tunnel: w760 -> [w799 _]
                      tunnel: [w799 0] -> w752
                      tunnel: w757 -> [_ _]
                      frame False {
                      }
                      frame True {
                      }
                    }
                    n369 = Not(x=w759) -> (.not. x?=w724:bool)
                    n370 = case shown="False" w727 {
                      tunnel: w725 -> [_ w792]
                      tunnel: [w788 w791] -> w723
                      tunnel: w724 -> [w788 _]
                      frame False {
                      }
                      frame True {
                        n371 = call "ProjectSearchDataName.vi"("element"="$Voltage Up") -> ("variant"=w797:variant)  [unwired: 7 in, 3 out]
                        n372 = call "ProjectSearchDataName.vi"("element"="$Voltage Dn") -> ("variant"=w796:variant)  [unwired: 7 in, 3 out]
                        n373 = Variant To Data(type=0.0, Variant=w797) -> (data=w794:dbl)  [unwired: 1 in, 1 out]
                        n374 = Variant To Data(type=0.0, Variant=w796) -> (data=w793:dbl)  [unwired: 1 in, 1 out]
                        n375 = In Range and Coerce(upper limit=w794, x=w792, lower limit=w793) -> (In Range?=w791:bool)  [unwired: 1 out]
                      }
                    }
                    n376 = Merge Errors(w744, w743) -> (w722:errorcluster)
                    n377 = Increment(x=w751) -> (x+1=w763:i32)
                    n378 = case shown="Error .." w722 {
                      tunnel: w723 -> [w764 _]
                      frame No Error {
                        n379 = case shown="True" w764 {
                          frame False {
                          }
                          frame True {
                            w765 = T13[] [enum."給PLC要量電壓訊號"] items=["S2站PC動作中_20", "電流量測完成產品OK_21", "電流量測完成產品NG_22", "S2站Format 執行_23", "S2 Format OK_24", "S2 Format NG_25", "S2站燒入執行_26", "S2站燒入OK_27", "S2站燒入NG_28", "S2站動作完成_29", "S3 PC動作中_30", "S3 Format 此站執行_31", "S3 Format OK_32", "S3 Format NG_33", "S3 燒入程式 此站執行_34", "S3 燒入程式 OK_35", "S3 燒入程式 NG_36", "S3 備用_37", "S3 備用_38", "S3 動作完成_39", "S4 PC動作中_40", "S4 量測完成 產品正常_41", "S4 量測完成 產品NG_42", "S4 Format 此站執行_43", "S4 Format OK_44", "S4 Format NG_45", "S4 燒入 此站不執行_46", "S4 燒入程式 OK_47", "S4 燒入程式 NG_48", "S4 藍芽Scan OK_49", "S4 藍芽Scan NG_50", "S4 動作完成_51", "給PLC要量電流訊號", "給PLC要量電壓訊號"]
                            w775 = T13[] [enum."S4 量測完成 產品正常_41"] items=["S2站PC動作中_20", "電流量測完成產品OK_21", "電流量測完成產品NG_22", "S2站Format 執行_23", "S2 Format OK_24", "S2 Format NG_25", "S2站燒入執行_26", "S2站燒入OK_27", "S2站燒入NG_28", "S2站動作完成_29", "S3 PC動作中_30", "S3 Format 此站執行_31", "S3 Format OK_32", "S3 Format NG_33", "S3 燒入程式 此站執行_34", "S3 燒入程式 OK_35", "S3 燒入程式 NG_36", "S3 備用_37", "S3 備用_38", "S3 動作完成_39", "S4 PC動作中_40", "S4 量測完成 產品正常_41", "S4 量測完成 產品NG_42", "S4 Format 此站執行_43", "S4 Format OK_44", "S4 Format NG_45", "S4 燒入 此站不執行_46", "S4 燒入程式 OK_47", "S4 燒入程式 NG_48", "S4 藍芽Scan OK_49", "S4 藍芽Scan NG_50", "S4 動作完成_51", "給PLC要量電流訊號", "給PLC要量電壓訊號"]
                            n380 = global read "Process Global.vi" "S4Tool Action"() -> (w768:bool[])
                            n381 = call "Set OutputPLC.vi"("Address In"=20, "Array 2"=w775, "Sat Coils"=bool[] [TRUE]) -> ("Error Out"=w771:errorcluster[])  [unwired: 7 in]
                            n382 = Replace Array Subset(array=w768, new element=TRUE ("new element/subarray"), index=5) -> (w769:bool[])
                            n383 = Merge Errors(w771) -> (w770:errorcluster)
                            n384 = global write "Process Global.vi" "S4Tool Action"(w769) -> ()
                            n385 = call "Set OutputPLC.vi"("Address In"=20, "Array 2"=w765, "Sat Coils"=bool[] [FALSE], "error in (no error)"=w770) -> ()  [unwired: 6 in, 1 out]
                          }
                        }
                      }
                      frame Error {
                        (unwired) bool[] [FALSE] ("Sat Coils")
                        w779 = T13[] [enum."給PLC要量電壓訊號"] items=["S2站PC動作中_20", "電流量測完成產品OK_21", "電流量測完成產品NG_22", "S2站Format 執行_23", "S2 Format OK_24", "S2 Format NG_25", "S2站燒入執行_26", "S2站燒入OK_27", "S2站燒入NG_28", "S2站動作完成_29", "S3 PC動作中_30", "S3 Format 此站執行_31", "S3 Format OK_32", "S3 Format NG_33", "S3 燒入程式 此站執行_34", "S3 燒入程式 OK_35", "S3 燒入程式 NG_36", "S3 備用_37", "S3 備用_38", "S3 動作完成_39", "S4 PC動作中_40", "S4 量測完成 產品正常_41", "S4 量測完成 產品NG_42", "S4 Format 此站執行_43", "S4 Format OK_44", "S4 Format NG_45", "S4 燒入 此站不執行_46", "S4 燒入程式 OK_47", "S4 燒入程式 NG_48", "S4 藍芽Scan OK_49", "S4 藍芽Scan NG_50", "S4 動作完成_51", "給PLC要量電流訊號", "給PLC要量電壓訊號"]
                        w787 = T13[] [enum."S4 量測完成 產品NG_42"] items=["S2站PC動作中_20", "電流量測完成產品OK_21", "電流量測完成產品NG_22", "S2站Format 執行_23", "S2 Format OK_24", "S2 Format NG_25", "S2站燒入執行_26", "S2站燒入OK_27", "S2站燒入NG_28", "S2站動作完成_29", "S3 PC動作中_30", "S3 Format 此站執行_31", "S3 Format OK_32", "S3 Format NG_33", "S3 燒入程式 此站執行_34", "S3 燒入程式 OK_35", "S3 燒入程式 NG_36", "S3 備用_37", "S3 備用_38", "S3 動作完成_39", "S4 PC動作中_40", "S4 量測完成 產品正常_41", "S4 量測完成 產品NG_42", "S4 Format 此站執行_43", "S4 Format OK_44", "S4 Format NG_45", "S4 燒入 此站不執行_46", "S4 燒入程式 OK_47", "S4 燒入程式 NG_48", "S4 藍芽Scan OK_49", "S4 藍芽Scan NG_50", "S4 動作完成_51", "給PLC要量電流訊號", "給PLC要量電壓訊號"]
                        n386 = global read "Process Global.vi" "S4Tool Action"() -> (w784:bool[])
                        n387 = call "Set OutputPLC.vi"("Address In"=20, "Array 2"=w787, "Sat Coils"=bool[] [TRUE]) -> ("Error Out"=w778:errorcluster[])  [unwired: 7 in]
                        n388 = Merge Errors(w778) -> (w777:errorcluster)
                        n389 = Replace Array Subset(array=w784, new element=FALSE ("new element/subarray"), index=5) -> (w785:bool[])
                        n390 = global write "Process Global.vi" "S4Tool Action"(w785) -> ()
                        n391 = call "Set OutputPLC.vi"("Address In"=20, "Array 2"=w779, "error in (no error)"=w777) -> ()  [unwired: 7 in, 1 out]
                      }
                    }
                    n392 = Select(t=w726, s=w723, f="NG" ("DataIn")) -> (s? t:f=w738:string)
                    n393 = Select(t=w763, s=w723, f=w751) -> (s? t:f=w750:i32)
                    n394 = global read "Main Glb.vi" "Input Registers0-99"() -> (w731:u16[])
                    n395 = call "Red PLC InReg.vi"("length"=10, "index"=40, "Input Registers Arr"=w731) -> ("Rad In Reg"=w732:string)  [unwired: 7 in, 1 out]
                    n396 = call "Cub Meaasure FGV.vi"("Action"=Table_Save."Write" ("Enum"), "Save Index"=MeasureDisplayTab."電池負載電壓", "DataIn"=w738, "SN"=w732) -> ()  [unwired: 8 in, 8 out]
                  }
                }
              }
            }
          }
          frame True {
          }
        }
        n397 = property class="DigNum (strict)"(reference=w25, "Value"=w26) -> ()  [unwired: 1 in, 2 out]
        n398 = disable-structure shown="Enabled" {
          disable-tunnel: w19 -> [w48 w51]
          disable-tunnel: [w47 w51] -> w20
          frame Disabled {
            n399 = call "ErrorCycleNoSet.vi"("error in"=w48, "CaseNo"=enum16{"S2", "S3", "S4", "S11"}."S4", "Error Set Item"="$AlarmCycleNo_S4") -> ("error out"=w47:errorcluster)  [unwired: 8 in]
          }
          frame Enabled {
          }
        }
        n400 = case shown="Error .." w19 {
          frame No Error {
            n401 = global write "Process Global.vi" "S4 OK"(TRUE ("S4 OK")) -> ()
          }
          frame Error {
            n402 = global write "Process Global.vi" "S4 NG"(TRUE ("S4 NG")) -> ()
          }
        }
        n403 = call "Exit.vi"("Enum"=enum16{"Initial", "Read", "Write"}."Read") -> ("ExitOut"=w22:bool)  [unwired: 10 in]
        n404 = Compound Arithmetic op=OR(w19, w31, w22) -> (w42:bool)
        "present" <- w30
      }
    }
    frame Error {
    }
  }
  n405 = disable-structure shown="Disabled" {
    frame Disabled {
      w815 = T14[] [enum."commamd1", enum."commamd2", enum."commamd3"] items=["Project Name", "commamd1", "commamd2", "commamd3", "wat time1", "return1", "return2", "return3", "wat time2", "over time", "retry"] ("Cmd Step")
      n406 = call "Project Cmd Combin.vi"("Cmd Step"=w815) -> ("concatenated string"=w814:string, "Content Input"=w816:string[])  [unwired: 7 in, 2 out]
      n407 = call "Tool RS232 test.vi"("Cmd In"=w814) -> ("error out"=w817:errorcluster, "action"=w808:u16)  [unwired: 8 in, 1 out]
      n408 = case shown="No Error" w817 {
        tunnel: [errorcluster {"status"=FALSE, "code"=0, "source"=""} ("error constant") errorcluster {"status"=TRUE, "code"=11500, "source"=""} ("error constant")] -> _
        frame No Error {
        }
        frame Error {
        }
      }
      n409 = Unbundle By Name(w817) -> ("status"=w809:bool)
      n410 = Not(x=w809) -> (.not. x?=w810:bool)
      n411 = Select(t=ProjectStepSelect."MToolWork" ("select step"), s=w810, f=ProjectStepSelect."Format" ("select step")) -> (s? t:f=w813:T12)
    }
    frame Enabled {
    }
  }
  n412 = disable-structure shown="Disabled" {
    frame Disabled {
      n413 = call "Scan Data Save.vi"() -> ()  [unwired: 11 in, 1 out]
    }
    frame Enabled {
    }
  }
  n414 = disable-structure shown="Disabled" {
    frame Disabled {
      n415 = global read "Main Glb.vi" "S4 Tary ID"() -> ()  [unwired: 1 in]
      n416 = global read "Main Glb.vi" "S4 Barcode ID"() -> ()  [unwired: 1 in]
    }
    frame Enabled {
    }
  }
  n417 = call "ErrorCycleNoSet.vi"("error in"=w2, "CaseNo"=enum16{"S2", "S3", "S4", "S11"}."S4", "Error Set Item"="$AlarmCycleNo_S4") -> ("error out"=w1:errorcluster)  [unwired: 8 in]
  "error out" <- w1
  n418 = disable-structure shown="Disabled" {
    disable-tunnel: w1 -> [w820 _]
    frame Disabled {
      n419 = case shown="Error .." w820 {
        frame No Error {
          n420 = global write "Process Global.vi" "S4 OK"(TRUE ("S4 OK")) -> ()
        }
        frame Error {
          n421 = global write "Process Global.vi" "S4 NG"(TRUE ("S4 NG")) -> ()
        }
      }
    }
    frame Enabled {
    }
  }
  n422 = Select(t=Station_Action."Dectect Action" ("Station Out"), s=w1, f=Station_Action."ImformOut" ("Station Out")) -> (s? t:f=→"Station Out":T1)
  "NG Pick out" <- "NG Pick in"
